vi "DetectorTest_MainV1.vi"() -> ()   [LabVIEW 2012]
uses:
  <vilib>/Analysis/NI_AALBase.lvlib
panel:
  in  "Move to 0 0":bool
  in  "Wafer Info Flash 2":T1={"Cell Name"="5500_130_05", "Package"="", "Coating"="", "LRC?"=enum."J2", "Comment"=""}
  in  "Parameters Flash 2":T2 {"Voc" format="%#_4g"; "Isc" format="%#_4g"; "FF" format="%#_4g"; "Imax" format="%#_4g"; "Vmax" format="%#_4g"; "Pmax" format="%#_4g"; "Itest" format="%#_4g"}
  in  "Wafer Info Flash":T1={"Cell Name"="5500_130_05", "Package"="", "Coating"="", "LRC?"=enum."J2", "Comment"=""}
  in  "Parameters Flash":T2 {"Voc" format="%#_4g"; "Isc" format="%#_4g"; "FF" format="%#_4g"; "Imax" format="%#_4g"; "Vmax" format="%#_4g"; "Pmax" format="%#_4g"; "Itest" format="%#_4g"}
  out "RawData file":path
  out "Fine Cell Clusters":T3(array[cluster])
  out "Selected Data":cluster{dbl[], dbl[]}
  in  "Test Results 2":T4
  in  "Session Info 2":T5={"V set"=-1.0, "I compliance"=0.001, "J set"=0.01, "I set"=0.0, "V compliance"=1.0, "Laser Power (mW)"=0.0, "TestID"=0, "Session Time"=timestamp(0 s since 1904-01-01), "Operator"="Radek"} {"V compliance" format="%#_6f"; "I compliance" format="%#_6e"}
  in  "Die Info 2":T6={"Device Name"="", "ActiveArea_um2"=3848.451, "MesaArea_um2"=3848.451, "x"=0.0, "y"=0.0}
  in  "Wafer Info 2":T7
  in  "Test Results":T4
  in  "Session Info":T5={"V set"=-1.0, "I compliance"=0.001, "J set"=0.01, "I set"=0.0, "V compliance"=1.0, "Laser Power (mW)"=0.0, "TestID"=0, "Session Time"=timestamp(0 s since 1904-01-01), "Operator"="Radek"} {"V compliance" format="%#_6f"; "I compliance" format="%#_6e"}
  in  "Die Info":T6={"Device Name"="", "ActiveArea_um2"=3848.451, "MesaArea_um2"=3848.451, "x"=0.0, "y"=0.0}
  in  "Wafer Info":T7
  in  "Name Array":string[](array[string])=["Wafer name", "Scribe", "Mask", "Lot", "Device name", "Active Area", "Mesa Area", "x", "y", "Imeas", "Vmeas", "Time", "Vset", "Icomp", "Jset", "Iset", "Vcomp", "Laser Power", "TestID", "SessionTime", "Operator", "Selected"]
  in  "TestID file":path=path "C:/Users/Flash/Desktop/LabVIEW/Detector IV/rawtest_log.csv"
  in  "update wafer":bool
  in  "Lot":string
  in  "Laser Power (mW)":dbl
  in  "Device Name":string
  in  "Scribe":string
  in  "MesaArea_um2":dbl=3848.451
  out "Status":string
  out "error out":errorcluster
  in  "error in (no error)":errorcluster
  out "Manaul Plot 1":cluster{"V manual":dbl[], dbl[]}[](array[cluster])
  out "Manual Plot 0":cluster{"V manual":dbl[], "I manual":dbl[]}[](array[cluster])
  in  "Reset 1st die":bool
  in  "Sweep Settings":T8={"Channel"=enum."Channel A", "Vstart"=-2.0, "Vend"=0.5, "# of points"=30, "NPLC"=1.0, "I compliance"=0.001, "Delay ms"=500.0}
  in  "Reset xy":bool
  out "current y":i32
  out "current x":i32
  in  "sweep delay ms":dbl=500.0
  in  "I compliance":dbl=0.001
  in  "points":u16=40
  in  "V end":dbl=0.4
  in  "V start":dbl=-1.5
  in  "Repeat Vf":u32=1
  out "I set":dbl
  in  "V compliance":dbl=1.0 format="%#_6f"
  in  "Vf delay ms":dbl=100.0
  in  "J set A/cm2":dbl=0.01
  in  "Repeat Id":u32=5
  in  "I compliance":dbl=0.001 format="%#_6e"
  in  "Id delay ms":dbl=500.0
  in  "V set":dbl=-1.0
  out "Vmeas Settings":T9={"Channel"=enum."Channel A", "Iset"=-1.0, "NPLC"=1.0, "V compliance"=0.001, "Repeat time"=3, "Delay ms"=500.0}
  out "Imeas Settings":T10={"Channel"=enum."Channel A", "Vset"=-1.0, "NPLC"=1.0, "I compliance"=0.001, "Repeat time"=3, "Delay ms"=500.0}
  out "Array of Cell Data Clusters":T11(array[cluster])=[{"Cell Name"="10000_590_4P5", "X-coord"=0.0, "Y-coord"=0.0, "Area"=110000000.0, "Grid Shadowing"=0.0081, "Ydim"=10000.0, "Xdim"=11000.0, "Meas Area"=0.0}, {"Cell Name"="10000_590_4P5", "X-coord"=10115.0, "Y-coord"=0.0, "Area"=110000000.0, "Grid Shadowing"=0.0081, "Ydim"=10000.0, "Xdim"=11000.0, "Meas Area"=0.0}, {"Cell Name"="10000_590_4P5", "X-coord"=20230.0, "Y-coord"=0.0, "Area"=110000000.0, "Grid Shadowing"=0.0081, "Ydim"=10000.0, "Xdim"=11000.0, "Meas Area"=0.0}, {"Cell Name"="10000_590_4P5", "X-coord"=30345.0, "Y-coord"=0.0, "Area"=110000000.0, "Grid Shadowing"=0.0081, "Ydim"=10000.0, "Xdim"=11000.0, "Meas Area"=0.0}, {"Cell Name"="10000_590_4P5", "X-coord"=-10115.0, "Y-coord"=11515.0, "Area"=110000000.0, "Grid Shadowing"=0.0081, "Ydim"=10000.0, "Xdim"=11000.0, "Meas Area"=0.0}, {"Cell Name"="10000_590_4P5", "X-coord"=0.0, "Y-coord"=11515.0, "Area"=110000000.0, "Grid Shadowing"=0.0081, "Ydim"=10000.0, "Xdim"=11000.0, "Meas Area"=0.0}, {"Cell Name"="10000_590_4P5", "X-coord"=10115.0, "Y-coord"=11515.0, "Area"=110000000.0, "Grid Shadowing"=0.0081, "Ydim"=10000.0, "Xdim"=11000.0, "Meas Area"=0.0}, {"Cell Name"="10000_590_4P5", "X-coord"=20230.0, "Y-coord"=11515.0, "Area"=110000000.0, "Grid Shadowing"=0.0081, "Ydim"=10000.0, "Xdim"=11000.0, "Meas Area"=0.0}, {"Cell Name"="10000_590_4P5", "X-coord"=30345.0, "Y-coord"=11515.0, "Area"=110000000.0, "Grid Shadowing"=0.0081, "Ydim"=10000.0, "Xdim"=11000.0, "Meas Area"=0.0}, {"Cell Name"="10000_590_4P5", "X-coord"=40460.0, "Y-coord"=11515.0, "Area"=110000000.0, "Grid Shadowing"=0.0081, "Ydim"=10000.0, "Xdim"=11000.0, "Meas Area"=0.0}, {"Cell Name"="10000_590_4P5", "X-coord"=-20230.0, "Y-coord"=23030.0, "Area"=110000000.0, "Grid Shadowing"=0.0081, "Ydim"=10000.0, "Xdim"=11000.0, "Meas Area"=0.0}, {"Cell Name"="10000_590_4P5", "X-coord"=-10115.0, "Y-coord"=23030.0, "Area"=110000000.0, "Grid Shadowing"=0.0081, "Ydim"=10000.0, "Xdim"=11000.0, "Meas Area"=0.0}, {"Cell Name"="10000_590_4P5", "X-coord"=0.0, "Y-coord"=23030.0, "Area"=110000000.0, "Grid Shadowing"=0.0081, "Ydim"=10000.0, "Xdim"=11000.0, "Meas Area"=0.0}, {"Cell Name"="10000_590_4P5", "X-coord"=10115.0, "Y-coord"=23030.0, "Area"=110000000.0, "Grid Shadowing"=0.0081, "Ydim"=10000.0, "Xdim"=11000.0, "Meas Area"=0.0}, {"Cell Name"="10000_590_4P5", "X-coord"=20230.0, "Y-coord"=23030.0, "Area"=110000000.0, "Grid Shadowing"=0.0081, "Ydim"=10000.0, "Xdim"=11000.0, "Meas Area"=0.0}, {"Cell Name"="10000_590_4P5", "X-coord"=30345.0, "Y-coord"=23030.0, "Area"=110000000.0, "Grid Shadowing"=0.0081, "Ydim"=10000.0, "Xdim"=11000.0, "Meas Area"=0.0}, {"Cell Name"="10000_590_4P5", "X-coord"=40460.0, "Y-coord"=23030.0, "Area"=110000000.0, "Grid Shadowing"=0.0081, "Ydim"=10000.0, "Xdim"=11000.0, "Meas Area"=0.0}, {"Cell Name"="10000_590_4P5", "X-coord"=50575.0, "Y-coord"=23030.0, "Area"=110000000.0, "Grid Shadowing"=0.0081, "Ydim"=10000.0, "Xdim"=11000.0, "Meas Area"=0.0}, {"Cell Name"="10000_590_4P5", "X-coord"=-20230.0, "Y-coord"=34545.0, "Area"=110000000.0, "Grid Shadowing"=0.0081, "Ydim"=10000.0, "Xdim"=11000.0, "Meas Area"=0.0}, {"Cell Name"="10000_590_4P5", "X-coord"=-10115.0, "Y-coord"=34545.0, "Area"=110000000.0, "Grid Shadowing"=0.0081, "Ydim"=10000.0, "Xdim"=11000.0, "Meas Area"=0.0}, {"Cell Name"="10000_590_4P5", "X-coord"=0.0, "Y-coord"=34545.0, "Area"=110000000.0, "Grid Shadowing"=0.0081, "Ydim"=10000.0, "Xdim"=11000.0, "Meas Area"=0.0}, {"Cell Name"="10000_590_4P5", "X-coord"=10115.0, "Y-coord"=34545.0, "Area"=110000000.0, "Grid Shadowing"=0.0081, "Ydim"=10000.0, "Xdim"=11000.0, "Meas Area"=0.0}, {"Cell Name"="10000_590_4P5", "X-coord"=20230.0, "Y-coord"=34545.0, "Area"=110000000.0, "Grid Shadowing"=0.0081, "Ydim"=10000.0, "Xdim"=11000.0, "Meas Area"=0.0}, {"Cell Name"="10000_590_4P5", "X-coord"=30345.0, "Y-coord"=34545.0, "Area"=110000000.0, "Grid Shadowing"=0.0081, "Ydim"=10000.0, "Xdim"=11000.0, "Meas Area"=0.0}, {"Cell Name"="10000_590_4P5", "X-coord"=40460.0, "Y-coord"=34545.0, "Area"=110000000.0, "Grid Shadowing"=0.0081, "Ydim"=10000.0, "Xdim"=11000.0, "Meas Area"=0.0}, {"Cell Name"="10000_590_4P5", "X-coord"=50575.0, "Y-coord"=34545.0, "Area"=110000000.0, "Grid Shadowing"=0.0081, "Ydim"=10000.0, "Xdim"=11000.0, "Meas Area"=0.0}, {"Cell Name"="10000_590_4P5", "X-coord"=-20230.0, "Y-coord"=46060.0, "Area"=110000000.0, "Grid Shadowing"=0.0081, "Ydim"=10000.0, "Xdim"=11000.0, "Meas Area"=0.0}, {"Cell Name"="10000_590_4P5", "X-coord"=-10115.0, "Y-coord"=46060.0, "Area"=110000000.0, "Grid Shadowing"=0.0081, "Ydim"=10000.0, "Xdim"=11000.0, "Meas Area"=0.0}, {"Cell Name"="10000_590_4P5", "X-coord"=0.0, "Y-coord"=46060.0, "Area"=110000000.0, "Grid Shadowing"=0.0081, "Ydim"=10000.0, "Xdim"=11000.0, "Meas Area"=0.0}, {"Cell Name"="10000_590_4P5", "X-coord"=10115.0, "Y-coord"=46060.0, "Area"=110000000.0, "Grid Shadowing"=0.0081, "Ydim"=10000.0, "Xdim"=11000.0, "Meas Area"=0.0}, {"Cell Name"="10000_590_4P5", "X-coord"=20230.0, "Y-coord"=46060.0, "Area"=110000000.0, "Grid Shadowing"=0.0081, "Ydim"=10000.0, "Xdim"=11000.0, "Meas Area"=0.0}, {"Cell Name"="10000_590_4P5", "X-coord"=30345.0, "Y-coord"=46060.0, "Area"=110000000.0, "Grid Shadowing"=0.0081, "Ydim"=10000.0, "Xdim"=11000.0, "Meas Area"=0.0}, {"Cell Name"="10000_590_4P5", "X-coord"=40460.0, "Y-coord"=46060.0, "Area"=110000000.0, "Grid Shadowing"=0.0081, "Ydim"=10000.0, "Xdim"=11000.0, "Meas Area"=0.0}, {"Cell Name"="10000_590_4P5", "X-coord"=50575.0, "Y-coord"=46060.0, "Area"=110000000.0, "Grid Shadowing"=0.0081, "Ydim"=10000.0, "Xdim"=11000.0, "Meas Area"=0.0}, {"Cell Name"="10000_590_4P5", "X-coord"=-10115.0, "Y-coord"=57575.0, "Area"=110000000.0, "Grid Shadowing"=0.0081, "Ydim"=10000.0, "Xdim"=11000.0, "Meas Area"=0.0}, {"Cell Name"="10000_590_4P5", "X-coord"=0.0, "Y-coord"=57575.0, "Area"=110000000.0, "Grid Shadowing"=0.0081, "Ydim"=10000.0, "Xdim"=11000.0, "Meas Area"=0.0}, {"Cell Name"="10000_590_4P5", "X-coord"=10115.0, "Y-coord"=57575.0, "Area"=110000000.0, "Grid Shadowing"=0.0081, "Ydim"=10000.0, "Xdim"=11000.0, "Meas Area"=0.0}, {"Cell Name"="10000_590_4P5", "X-coord"=20230.0, "Y-coord"=57575.0, "Area"=110000000.0, "Grid Shadowing"=0.0081, "Ydim"=10000.0, "Xdim"=11000.0, "Meas Area"=0.0}, {"Cell Name"="10000_590_4P5", "X-coord"=30345.0, "Y-coord"=57575.0, "Area"=110000000.0, "Grid Shadowing"=0.0081, "Ydim"=10000.0, "Xdim"=11000.0, "Meas Area"=0.0}, {"Cell Name"="10000_590_4P5", "X-coord"=40460.0, "Y-coord"=57575.0, "Area"=110000000.0, "Grid Shadowing"=0.0081, "Ydim"=10000.0, "Xdim"=11000.0, "Meas Area"=0.0}, {"Cell Name"="10000_590_4P5", "X-coord"=0.0, "Y-coord"=69090.0, "Area"=110000000.0, "Grid Shadowing"=0.0081, "Ydim"=10000.0, "Xdim"=11000.0, "Meas Area"=0.0}, {"Cell Name"="10000_590_4P5", "X-coord"=10115.0, "Y-coord"=69090.0, "Area"=110000000.0, "Grid Shadowing"=0.0081, "Ydim"=10000.0, "Xdim"=11000.0, "Meas Area"=0.0}, {"Cell Name"="10000_590_4P5", "X-coord"=20230.0, "Y-coord"=69090.0, "Area"=110000000.0, "Grid Shadowing"=0.0081, "Ydim"=10000.0, "Xdim"=11000.0, "Meas Area"=0.0}, {"Cell Name"="10000_590_4P5", "X-coord"=30345.0, "Y-coord"=69090.0, "Area"=110000000.0, "Grid Shadowing"=0.0081, "Ydim"=10000.0, "Xdim"=11000.0, "Meas Area"=0.0}]
  in  "stop":bool
  in  "ActiveArea_um2":dbl=3848.451
  in  "NPLC":dbl=1.0
  in  "Operator":string(combo)="Radek"
  in  "Mask":string
  in  "Wafer Name":string
  in  "Tab Control":T12(tab)
  in  "Manual_Test":bool
  in  "Manual IV settting":enum32{"Linear plot", "Log plot"}(radio)
  out "Vmeas manual":dbl
  out "Imeas manual":dbl
  out "Iarray manual":dbl[](array[numeric])
  out "Varray manual":dbl[](array[numeric])
  out "y target":i32
  out "x target":i32
  in  "Die Number":u16(ring) items=["0", "1", "2", "3", "4", "5", "6", "7", "8", "9"]
  in  "load file":bool
  in  "Move to":bool
  in  "Mask File Manual":path=path "C:/Users/Flash/Desktop/Mask Files/SL066 Detector/SL066_D5_20_align on D3000.csv"
  out "Manual IV":cluster{"V manual":dbl[], "I manual":dbl[]}[](graph)
  in  "Load raw":bool
  in  "Select":bool
  in  "Number Select":u16=10
  in  "Vmax":dbl=0.95
  in  "Vmin":dbl
  out "Test FileName":string
  out "RawTest ID":u32
  out "Progress":u8(slide) scale=0.0..100.0
  out "Current Device":u32
  out "Total Device":u32
  out "V meas":dbl[](array[numeric])
  out "I meas":dbl[](array[numeric])
  in  "RawData Save Path":path=path "C:/Users/Flash/Desktop/Data/Detector test data"
  in  "StartRaw":bool
  out "Vforward hist":T13(graph)
  out "Idark hist":T13(graph)
  in  "Mask File Raw":path=path "C:/Users/Flash/Desktop/Mask Files/SL066 Detector/SL066_D5_20_align on D3000.csv"
  out "Spec Plot":cluster{"V meas":dbl[], "I meas":dbl[]}[](graph)
  in  "Auto Select and Fine Test?":bool
  in  "FineTest save path":path=path "C:/Users/Flash/Desktop/Data/Detector test data/IV"
  out "I fine":dbl[](array[numeric])
  out "V fine":dbl[](array[numeric])
  out "Current Device":u32
  out "Total Device":u32
  out "IV fine log":cluster{dbl[], dbl[]}[](graph)
  out "Progress 2":u8(slide) scale=0.0..100.0
  in  "StartFine":bool
  out "IV fine linear":cluster{dbl[], dbl[]}[](graph)
  in  "Mask File Fine":path=path "C:/Users/Flash/Desktop/Mask Files/SL066 Detector/SL066_D5_20_align on D3000.csv"
  in  "Prober GPIB":string="0:1"
  in  "SMU":refnum<visa-resource-name>="GPIB0::26::INSTR"
  in  "Channel":enum32{"Channel A", "Channel B"}(ring)
  # "0 is for dark IV!"
  # "Sweep Settings"
  # "Forward Voltage"
  # "Dark/Light Current"
  # "Make sure current x and y are same as prober before click Start!"
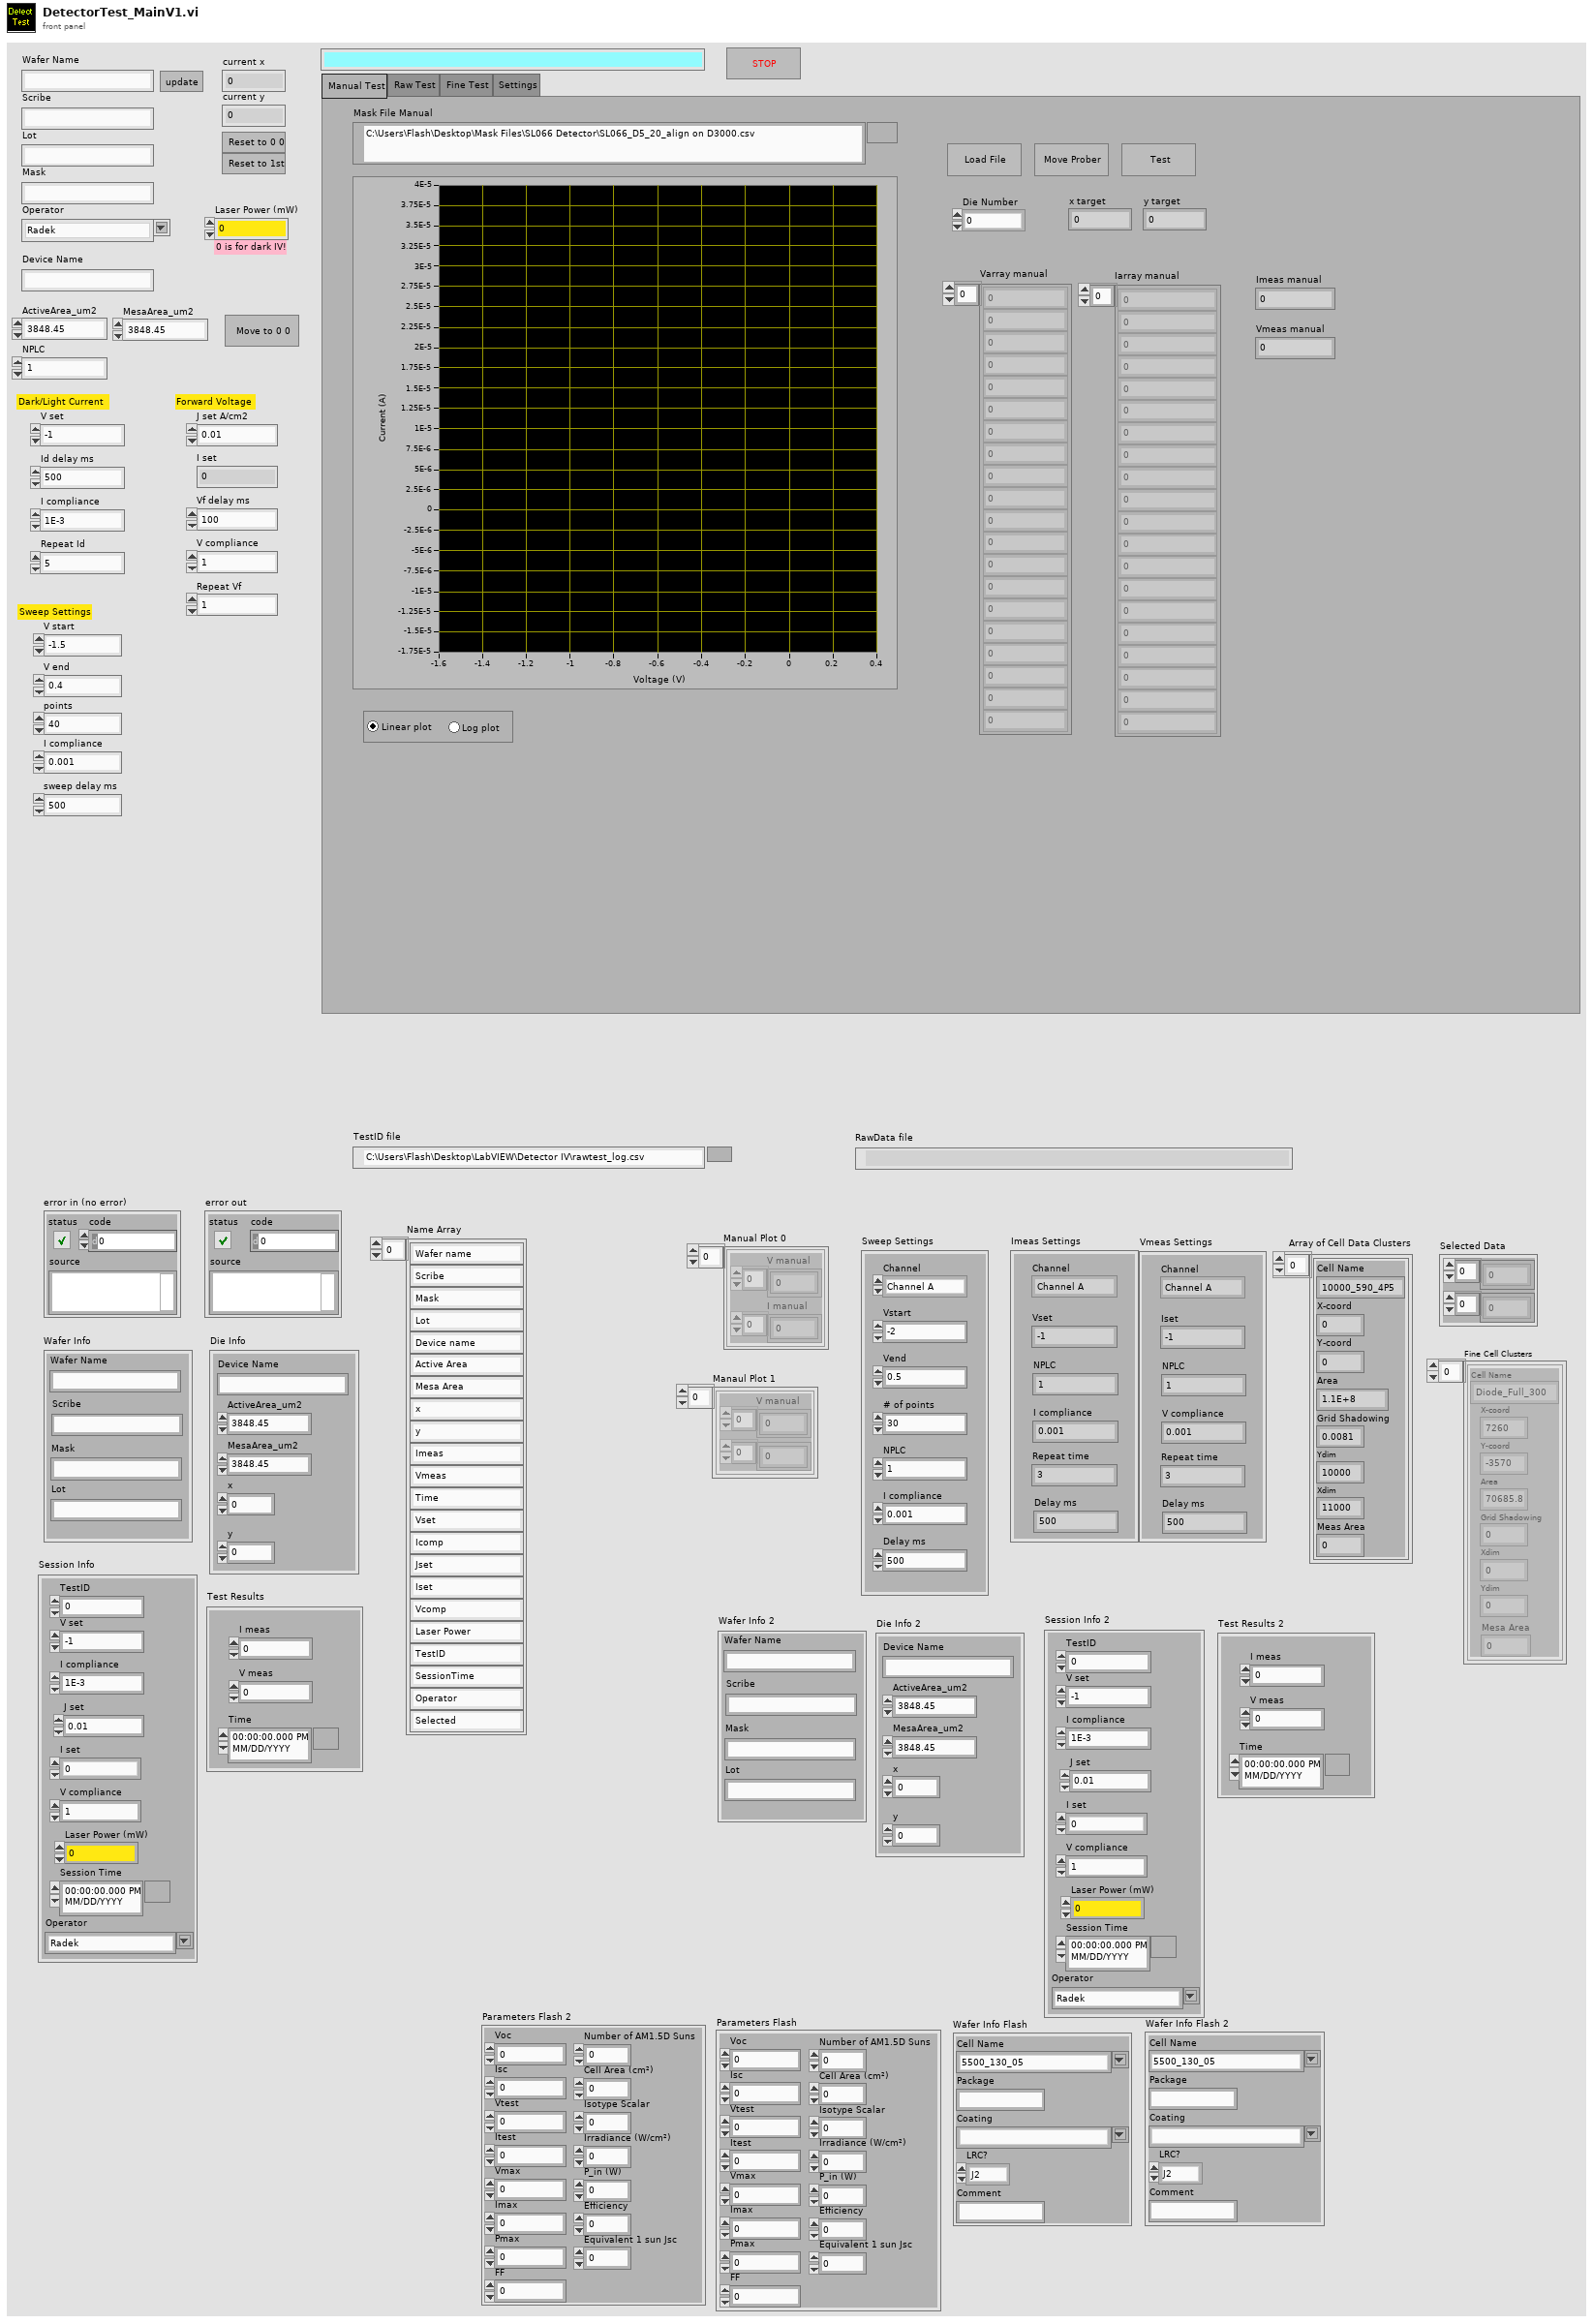
[diagram p1: front panel]
types:
  T1 = cluster{"Cell Name":string, "Package":string, "Coating":string, "LRC?":enum16{"J1", "J2", "LRC"}, "Comment":string}
  T2 = cluster{"Voc":dbl, "Isc":dbl, "FF":dbl, "Vtest":dbl, "Imax":dbl, "Vmax":dbl, "Pmax":dbl, "Itest":dbl, "Efficiency":dbl, "P_in (W)":dbl, "Irradiance (W/cm²)":dbl, "Cell Area (cm²)":dbl, "Number of AM1.5D Suns":dbl, "Isotype Scalar":dbl, "Equivalent 1 sun Jsc":dbl}
  T3 = cluster{"Cell Name":string, "X-coord":dbl, "Y-coord":dbl, "Area":dbl, "Grid Shadowing":dbl, "Xdim":dbl, "Ydim":dbl, "Mesa Area":dbl}[]
  T4 = cluster{"I meas":dbl, "V meas":dbl, "Time":timestamp}
  T5 = cluster{"V set":dbl, "I compliance":dbl, "J set":dbl, "I set":dbl, "V compliance":dbl, "Laser Power (mW)":dbl, "TestID":u32, "Session Time":timestamp, "Operator":string}
  T6 = cluster{"Device Name":string, "ActiveArea_um2":dbl, "MesaArea_um2":dbl, "x":dbl, "y":dbl}
  T7 = cluster{"Wafer Name":string, "Scribe":string, "Mask":string, "Lot":string}
  T8 = cluster{"Channel":enum32{"Channel A", "Channel B"}, "Vstart":dbl, "Vend":dbl, "# of points":u16, "NPLC":dbl, "I compliance":dbl, "Delay ms":dbl}
  T9 = cluster{"Channel":enum32{"Channel A", "Channel B"}, "Iset":dbl, "NPLC":dbl, "V compliance":dbl, "Repeat time":u16, "Delay ms":dbl}
  T10 = cluster{"Channel":enum32{"Channel A", "Channel B"}, "Vset":dbl, "NPLC":dbl, "I compliance":dbl, "Repeat time":u16, "Delay ms":dbl}
  T11 = cluster{"Cell Name":string, "X-coord":dbl, "Y-coord":dbl, "Area":dbl, "Grid Shadowing":dbl, "Ydim":dbl, "Xdim":dbl, "Meas Area":dbl}[]
  T12 = enum32{"Manual Test", "Raw Test", "Fine Test", "Settings"}
  T13 = cluster{"X Values":dbl[], "Histogram: h(x)":i32[]}
  T14 = cluster{"Cell Name":string, "X-coord":dbl, "Y-coord":dbl, "Area":dbl, "Grid Shadowing":dbl, "Ydim":dbl, "Xdim":dbl, "Meas Area":dbl}
  T15 = cluster{"Varray manual":dbl[], "Iarray manual":dbl[]}[]
  T16 = cluster{"WaferName":string, "Scribe":string, "Structure":string, "Lot":string, "Mask":string}
  T17 = cluster{"V set":dbl, "I compliance":dbl, "J set":dbl, "I set":dbl, "V compliance":dbl, "Laser Power (mW)":dbl, "TestID":u32, "Operator":string}
  T18 = cluster{"Device Name":string, "ActiveArea_um2":dbl, "MesaArea_um2":dbl}
  T19 = cluster{"Cell Name":string, "X-coord":dbl, "Y-coord":dbl, "Area":dbl, "Grid Shadowing":dbl, "Xdim":dbl, "Ydim":dbl, "Mesa Area":dbl}
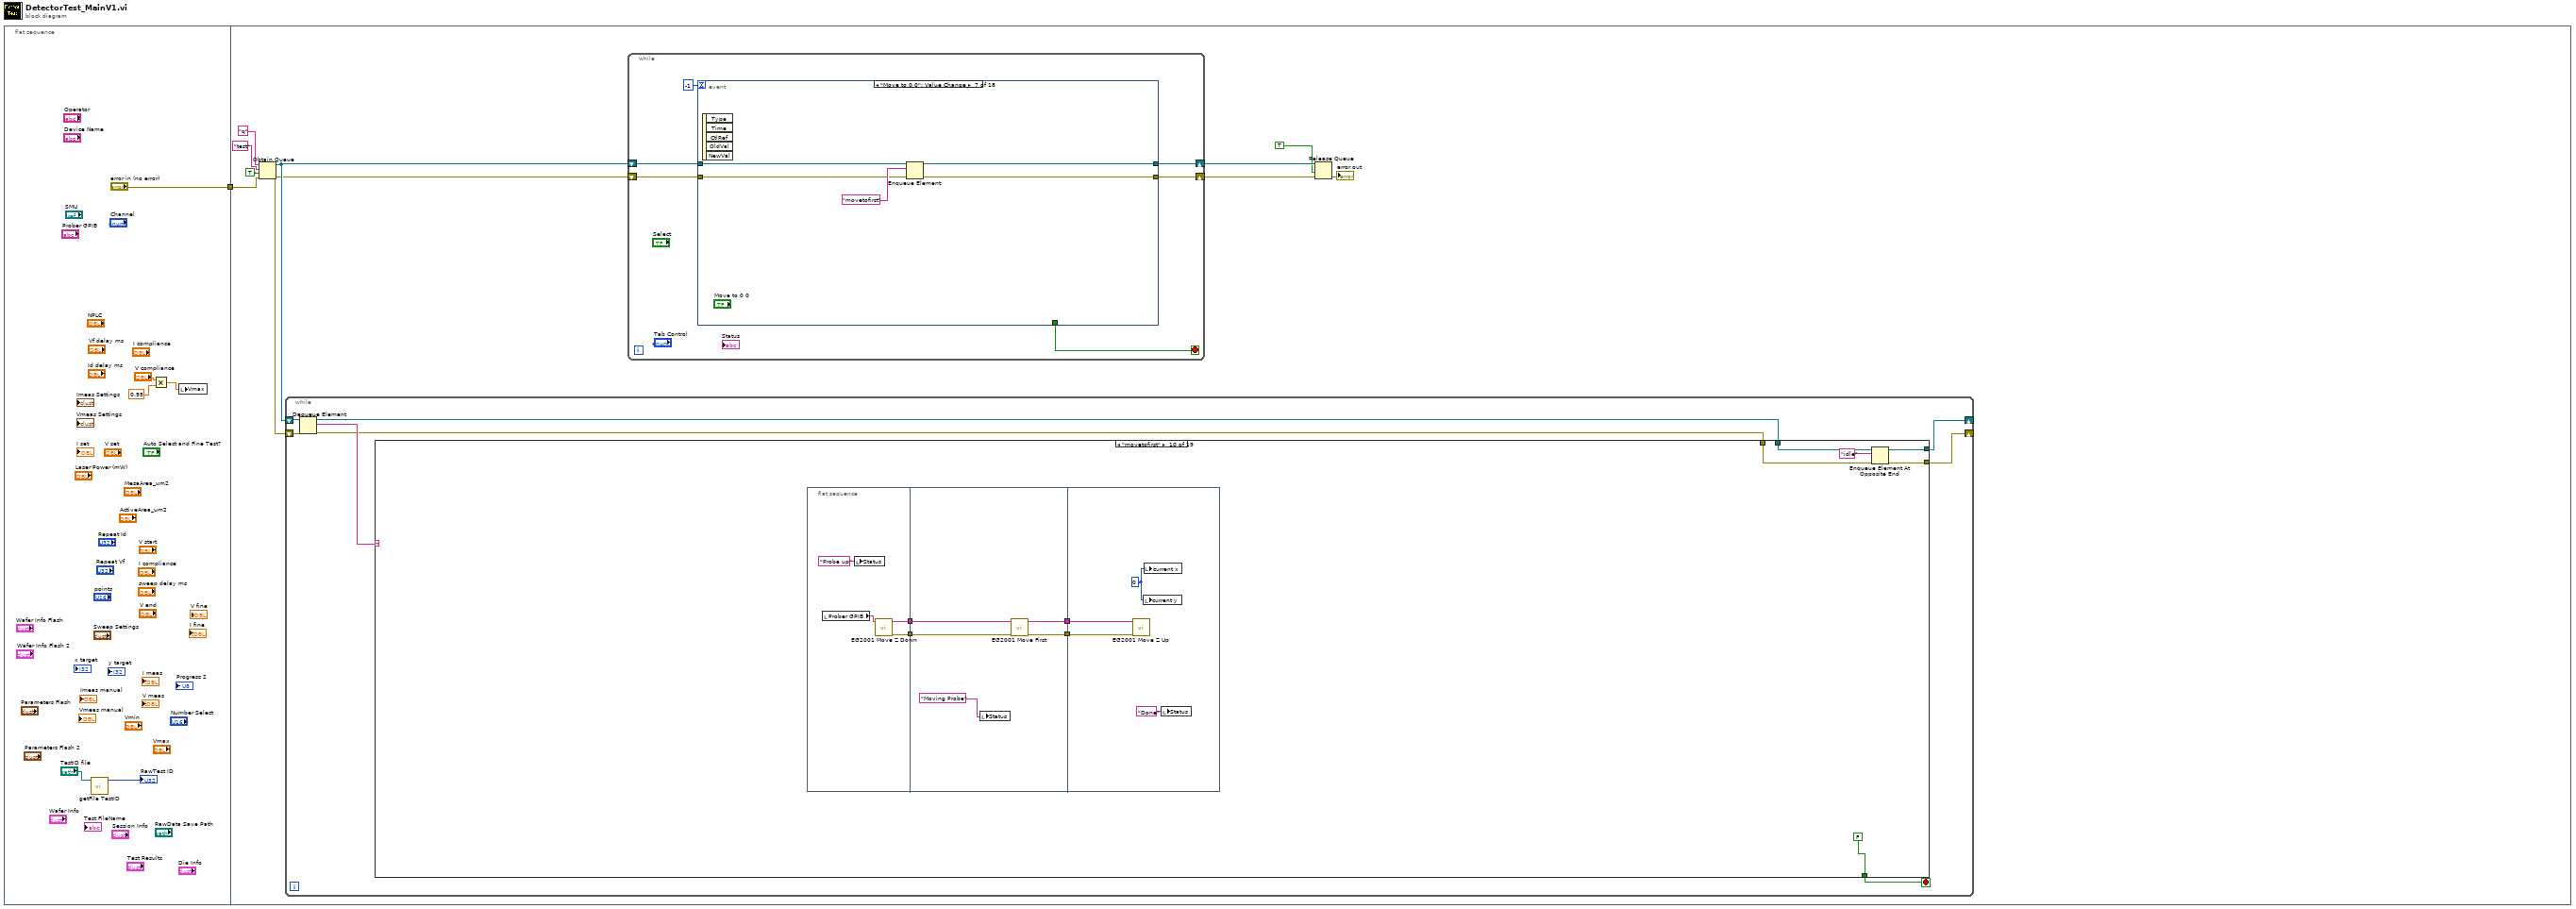
[diagram p0: block diagram]
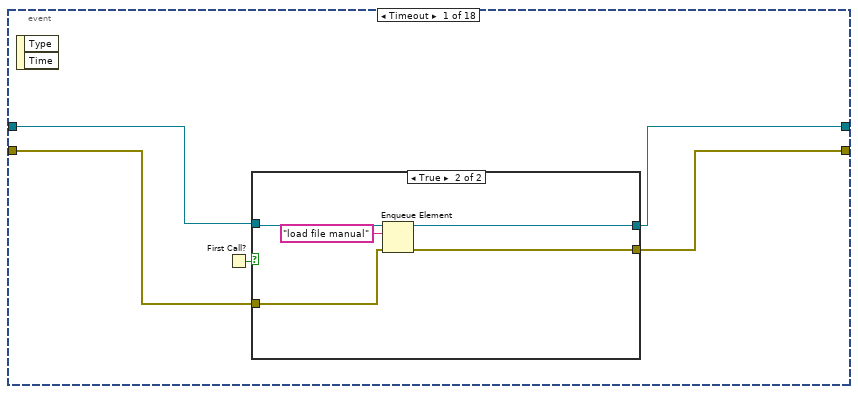
[diagram p2: hidden frame]
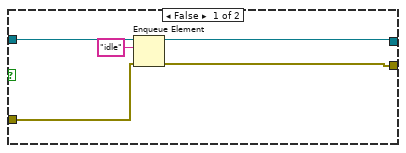
[diagram p3: hidden frame]
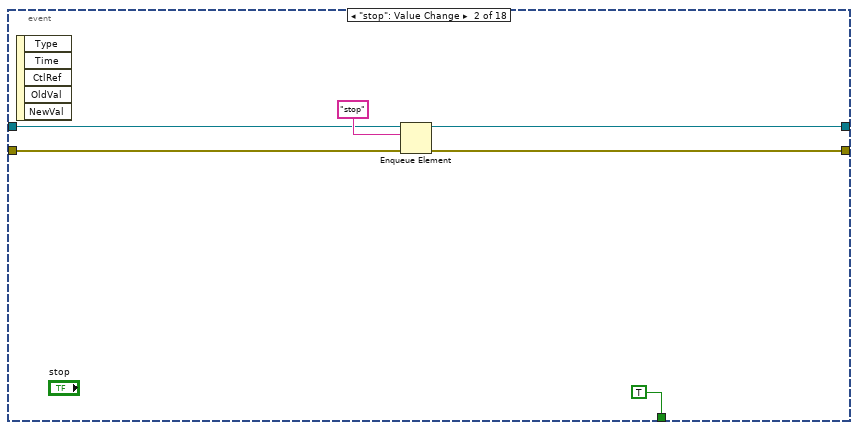
[diagram p4: hidden frame]
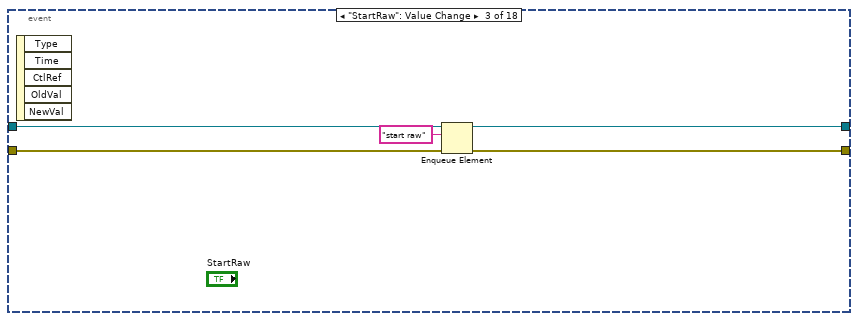
[diagram p5: hidden frame]
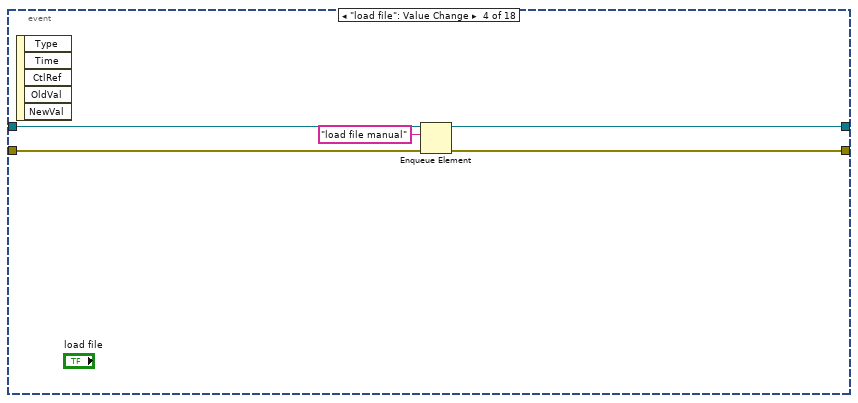
[diagram p6: hidden frame]
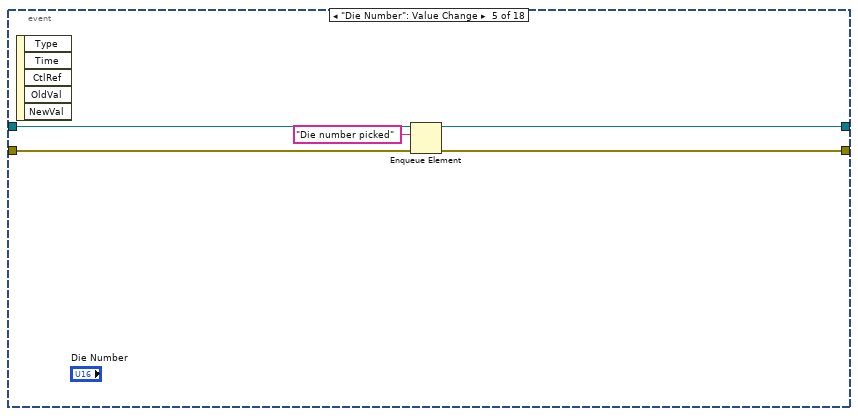
[diagram p7: hidden frame]
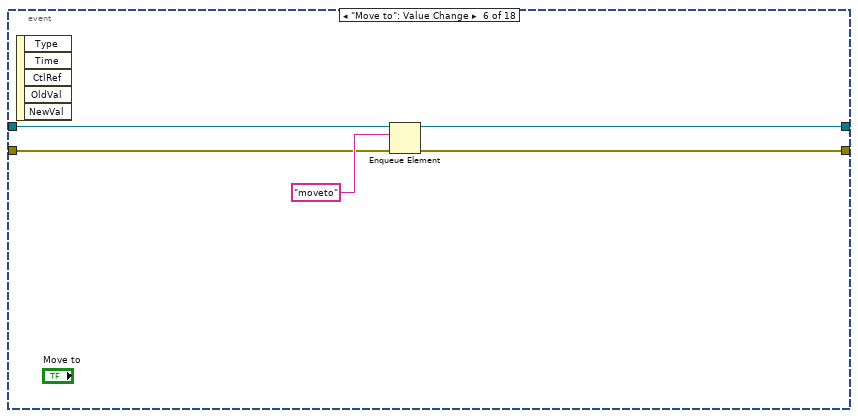
[diagram p8: hidden frame]
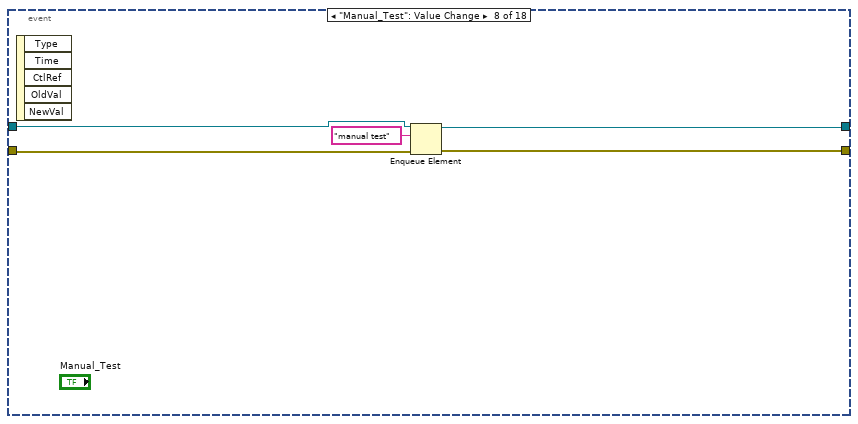
[diagram p9: hidden frame]
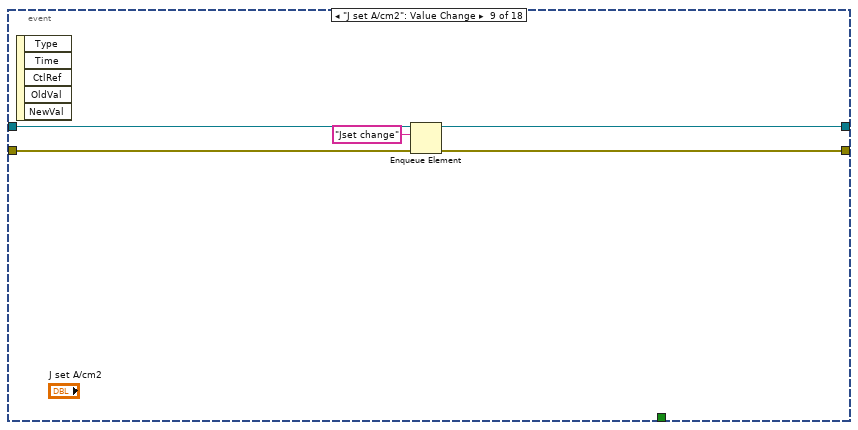
[diagram p10: hidden frame]
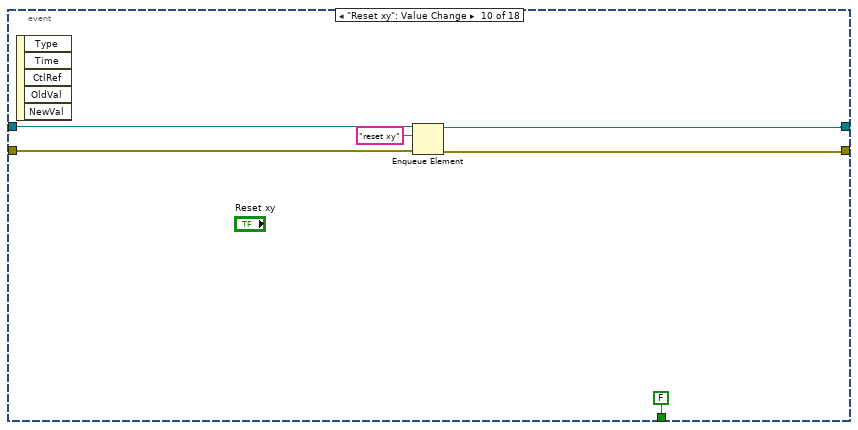
[diagram p11: hidden frame]
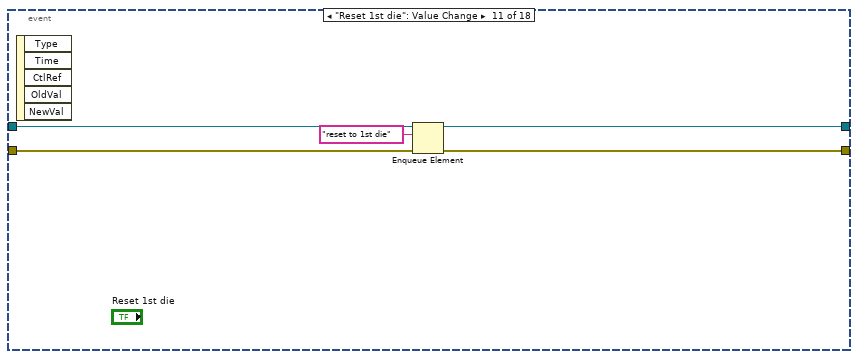
[diagram p12: hidden frame]
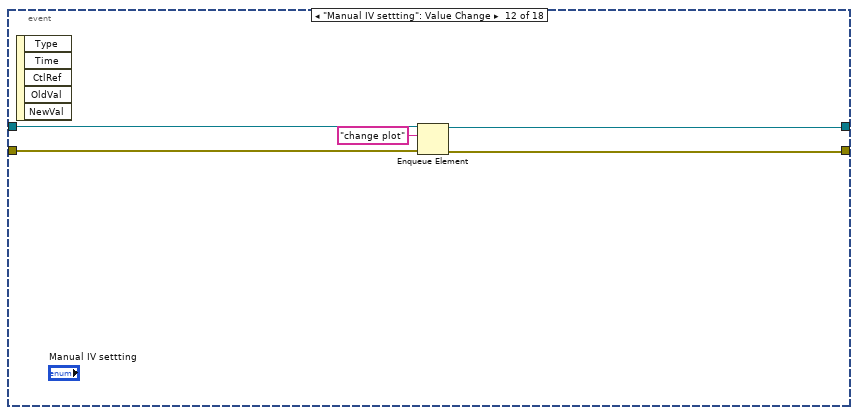
[diagram p13: hidden frame]
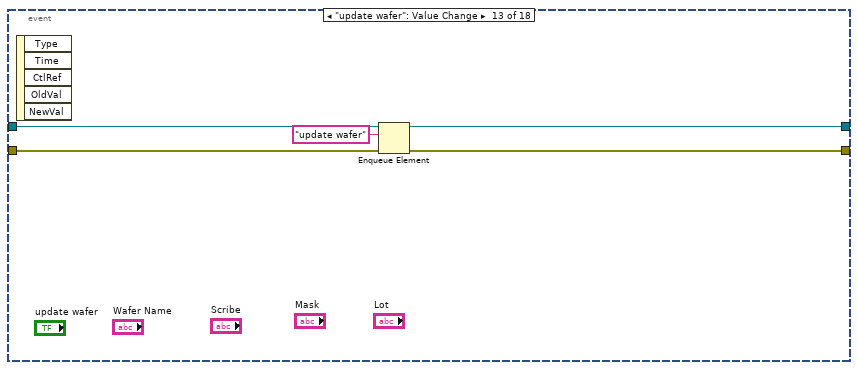
[diagram p14: hidden frame]
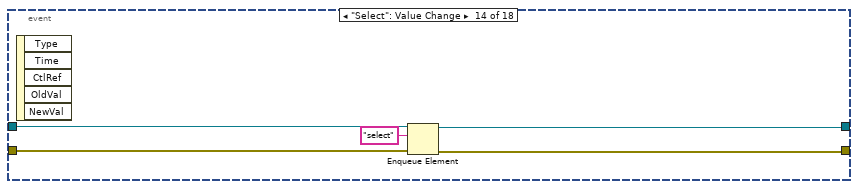
[diagram p15: hidden frame]
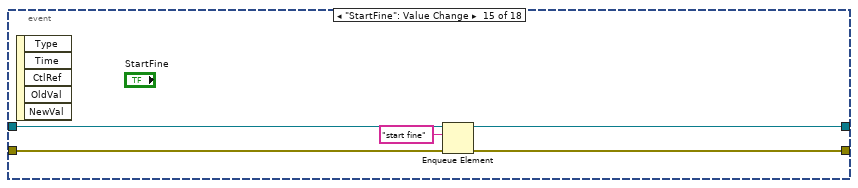
[diagram p16: hidden frame]
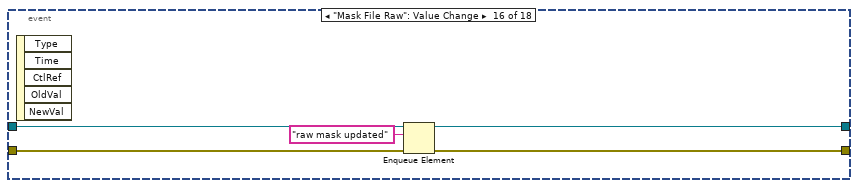
[diagram p17: hidden frame]
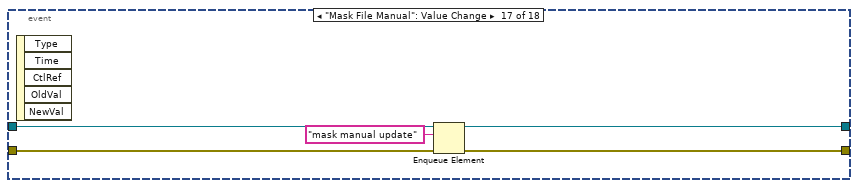
[diagram p18: hidden frame]
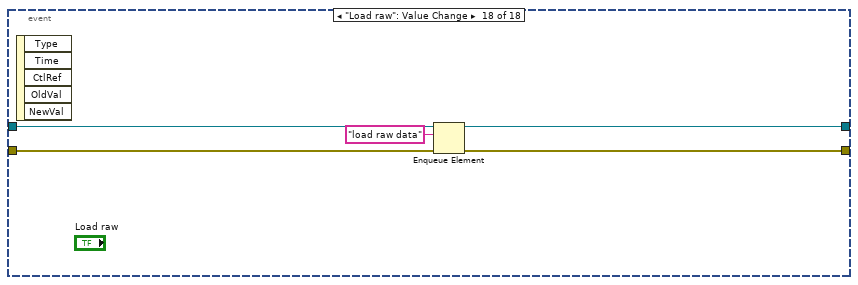
[diagram p19: hidden frame]
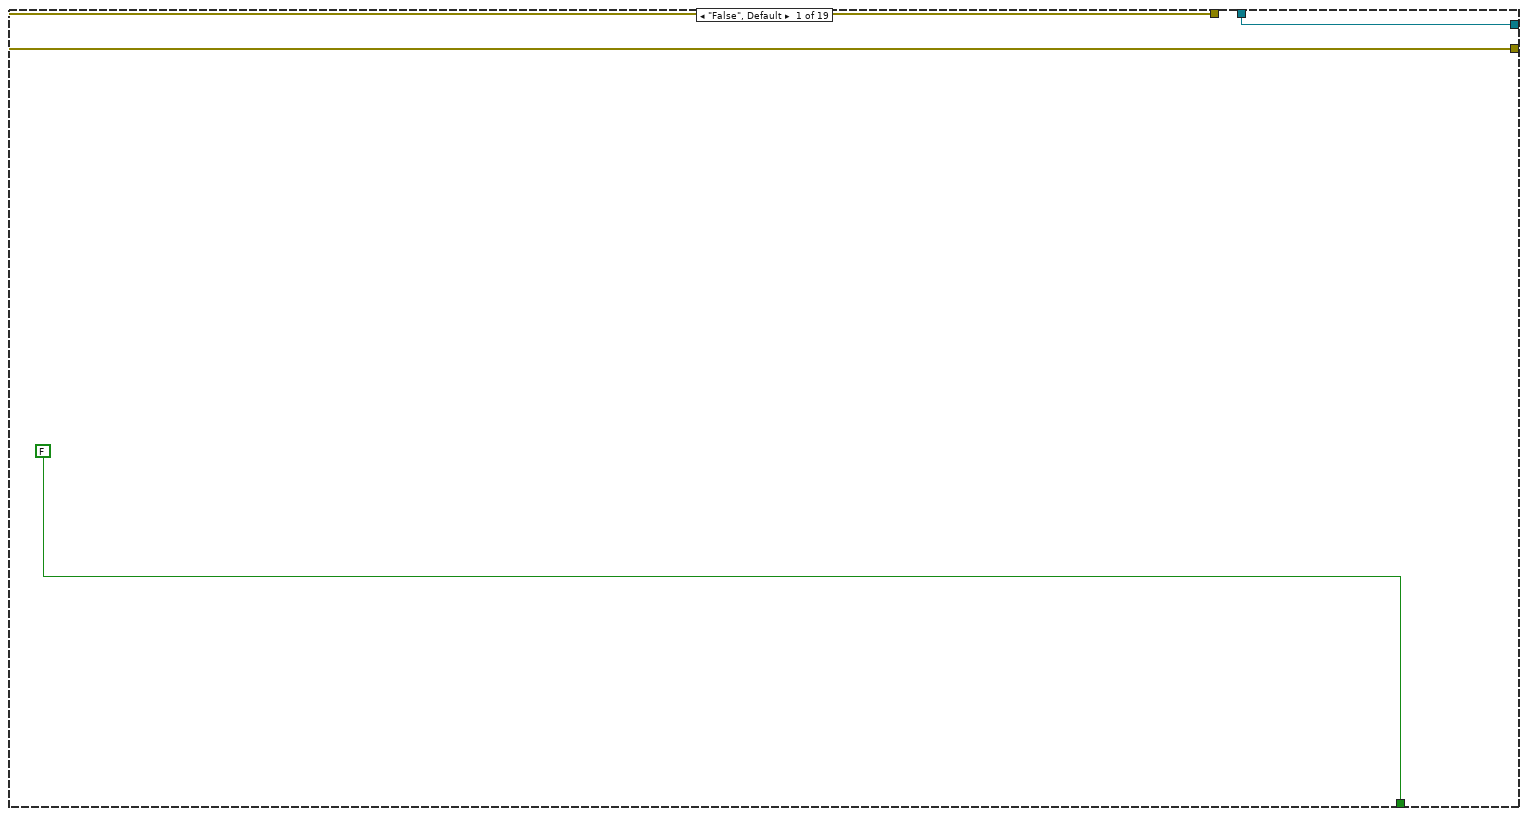
[diagram p20: hidden frame]
diagram:
  n1 = flat-sequence {
    tunnel: ["error in (no error)"] -> w1
    tunnel: w1 -> [w14]
    frame #0 {
      n2 = call "getFile TestID.vi"("Path"="TestID file") -> ("TestID"=→"RawTest ID":u32)  [unwired: 9 in, 1 out]
      n3 = Multiply(x="V compliance", y=0.95) -> (x*y=w2:dbl)
      n4 = local write "Vmax"(w2) -> ()
    }
    frame #1 {
      n5 = Obtain Queue(name (unnamed)="q", element data type="test" ("name (unnamed)"), create if not found? (T)=TRUE, error in (no error)=w14) -> (queue out=w16:refnum<queue>, error out=w15:errorcluster)  [unwired: 1 in, 1 out]
      n6 = while {
        shift-right: [w131] -> _
        shift-left: w16 -> [w128]
        shift-right: [w130] -> _
        shift-left: w15 -> [w127]
        stop <- w133 stop-if-true
        n7 = Dequeue Element(queue=w128, error in (no error)=w127) -> (queue out=w126:refnum<queue>, element=w132:string, error out=w129:errorcluster)  [unwired: 1 in, 1 out]
        n8 = case shown="\"movetofirst\"" w132 {
          tunnel: [FALSE TRUE FALSE FALSE FALSE FALSE FALSE FALSE FALSE FALSE FALSE FALSE FALSE FALSE FALSE FALSE FALSE FALSE FALSE] -> w133
          tunnel: w129 -> [w135 w138 w143 w303 w314 w325 w356 w380 w393 w425 w450 w530 w540 w547 w562 w597 w634 w775 w786]
          tunnel: [w135 w138 w144 w304 w311 w322 w359 w381 w396 w428 w449 w535 w540 w546 w564 w599 w636 w777 w788] -> w130
          tunnel: w126 -> [w134 w137 w146 w306 w313 w324 w357 w383 w398 w430 w447 w537 w541 w545 w563 w598 w635 w776 w787]
          tunnel: [w134 w137 w145 w305 w312 w323 w358 w382 w397 w429 w448 w536 w541 w544 w565 w600 w637 w778 w789] -> w131
          frame "False", Default {
          }
          frame "stop" {
          }
          frame "start raw" {
            n9 = flat-sequence {
              tunnel: [w157] -> w142
              tunnel: w142 -> [w187]
              tunnel: [w187] -> w141
              tunnel: [w177] -> w140
              tunnel: w141 -> [w189]
              tunnel: w140 -> [w188]
              frame #0 {
                n10 = local read "Wafer Name"() -> (w155:string)
                n11 = local read "RawTest ID"() -> (w160:u32)
                n12 = local read "Scribe"() -> (w154:string)
                n13 = local read "Mask"() -> (w153:string)
                n14 = local read "Lot"() -> (w152:string)
                n15 = call "Device Files v1.vi"("Rows"=1200, "Mask file path"="Mask File Raw") -> ("size(s)"=w157:i32, "Array of Cell Clusters"=→"Array of Cell Data Clusters":T3)  [unwired: 6 in, 2 out]
                "Total Device" <- w157
                n16 = Increment(x=w160) -> (x+1=w159:u32)
                n17 = Bundle By Name(cluster="Wafer Info 2", "Wafer Name"=w155, "Scribe"=w154, "Mask"=w153, "Lot"=w152) -> (w156:T7)
                n18 = local write "Status"("Prepare raw test" ("Status")) -> ()
                n19 = Initialize Array(nan ("element"), w157) -> (w150:dbl[])
                n20 = local write "RawTest ID"(w159) -> ()
                n21 = Bundle(w150, w150) -> (→"Selected Data":cluster{dbl[], dbl[]})  [unwired: 1 in]
                n22 = local write "Wafer Info"(w156) -> ()
                n23 = local write "V meas"(w150) -> ()
                n24 = local write "I meas"(w150) -> ()
                "Progress" <- u8 0 ("Progress")
              }
              frame #1 {
                n25 = local read "Laser Power (mW)"() -> (w168:dbl)
                n26 = local read "V compliance"() -> (w169:dbl)
                n27 = local read "RawData Save Path"() -> (w181:path)
                n28 = local read "I compliance"() -> (w172:dbl)
                n29 = local read "RawTest ID"() -> (w167:u32)
                n30 = local read "Array of Cell Data Clusters"() -> (w186:T11)
                n31 = local read "Operator"() -> (w166:string)
                n32 = local read "J set A/cm2"() -> (w171:dbl)
                n33 = local read "Wafer Name"() -> (w183:string)
                n34 = local read "V set"() -> (w173:dbl)
                n35 = local read "I set"() -> (w170:dbl)
                n36 = Index Array(array=w186, index=0) -> (element=w184:T14)
                n37 = Unbundle By Name(w184) -> ("Cell Name"=w182:string)
                n38 = call "get RawTest filename.vi"("Device Name"=w182, "Wafer Name"=w183) -> ("current time"=w174:timestamp, "FileName"=w180:string)  [unwired: 8 in]
                n39 = Build Path(base path=w181, name or relative path=w180) -> (appended path=w179:path)
                n40 = local write "Test FileName"(w180) -> ()
                n41 = Bundle By Name(cluster="Session Info 2", "V set"=w173, "I compliance"=w172, "J set"=w171, "I set"=w170, "V compliance"=w169, "Laser Power (mW)"=w168, "TestID"=w167, "Session Time"=w174, "Operator"=w166) -> (w175:T5)
                n42 = call "writeFile RawTestHead.vi"("Name Array"="Name Array", "Path"=w179) -> ("Path out"=w177:path)  [unwired: 9 in]
                "RawData file" <- w177
                n43 = local write "Session Info"(w175) -> ()
              }
              frame #2 {
                n44 = for {
                  N: w189 -> [w202]
                  tunnel: w188 -> [w190]
                  i -> [w191]
                  n45 = flat-sequence {
                    tunnel: [w237] -> w212
                    tunnel: [w236] -> w211
                    tunnel: w191 -> [w230]
                    tunnel: [w232] -> w206
                    tunnel: [w231] -> w205
                    tunnel: [w214] -> w204
                    tunnel: [w213] -> w203
                    tunnel: w212 -> [w238]
                    tunnel: w211 -> [w246]
                    tunnel: [w245] -> w210
                    tunnel: [w244] -> w209
                    tunnel: w206 -> [w242]
                    tunnel: w205 -> [w241]
                    tunnel: w204 -> [w240]
                    tunnel: w203 -> [w239]
                    tunnel: w210 -> [w249]
                    tunnel: w209 -> [w248]
                    tunnel: [w259] -> w208
                    tunnel: [w258] -> w207
                    tunnel: w208 -> [w262]
                    tunnel: w207 -> [w270]
                    tunnel: [w262] -> w193
                    tunnel: [w263] -> w192
                    tunnel: w193 -> [w281]
                    tunnel: w192 -> [w280]
                    tunnel: w191 -> [w287]
                    tunnel: w190 -> [w278]
                    frame #0 {
                      n46 = local read "Array of Cell Data Clusters"() -> (w234:T11)
                      n47 = local read "Device Name"() -> (w217:string)
                      n48 = Increment(x=w230) -> (x+1=→"Current Device":i32)
                      n49 = local read "Laser Power (mW)"() -> (w226:dbl)
                      n50 = Index Array(array=w234, index=w230) -> (element=w227:T14)
                      n51 = local read "Prober GPIB"() -> (w228:string)
                      n52 = Unbundle By Name(w227) -> ("X-coord"=w214:dbl, "Y-coord"=w213:dbl, "Area"=w215:dbl, "Meas Area"=w216:dbl, "Cell Name"=w220:string)
                      n53 = Bundle By Name(cluster="Die Info 2", "Device Name"=w217, "ActiveArea_um2"=w215, "MesaArea_um2"=w216, "x"=w214, "y"=w213) -> (w218:T6)
                      n54 = call "get Area.vi"("Laser"=w226, "Cell Data Cluster"=w227) -> ("Area"=w224:dbl)  [unwired: 9 in]
                      n55 = local read "J set A/cm2"() -> (w222:dbl)
                      n56 = local write "ActiveArea_um2"(w215) -> ()
                      n57 = local write "MesaArea_um2"(w216) -> ()
                      n58 = local write "Device Name"(w220) -> ()
                      n59 = Divide(x=w224, y=100000000.0) -> (x/y=w223:dbl)
                      n60 = local read "current y"() -> (w233:i32)
                      n61 = call "EG2001 Move Z Down.vi"("GPIB Address"=w228) -> ("Error Out"=w236:errorcluster, "GPIB Address Out"=w237:string)  [unwired: 9 in]
                      n62 = local read "current x"() -> (w235:i32)
                      n63 = local write "Die Info"(w218) -> ()
                      n64 = Multiply(x=w222, y=w223) -> (x*y=w221:dbl)
                      n65 = local write "I set"(w221) -> ()
                      n66 = Subtract(x=w214, y=w235) -> (x-y=w232:dbl)
                      n67 = Subtract(x=w213, y=w233) -> (x-y=w231:dbl)
                    }
                    frame #1 {
                      n68 = local write "current x"(w240) -> ()
                      n69 = local write "current y"(w239) -> ()
                      n70 = call "EG2001 Move Machine Step X-Y.vi"("Flip X Coordinates?"=FALSE, "Y"=w241, "Steps/Microns"=enum32{"Steps", "Microns"}."Microns", "X"=w242, "error in (no error)"=w246, "GPIB Address"=w238) -> ("Error Out"=w244:errorcluster, "GPIB Address Out"=w245:string)  [unwired: 4 in]
                    }
                    frame #2 {
                      n71 = call "EG2001 Move Z Up.vi"("error in (no error)"=w248, "GPIB Address"=w249) -> ()  [unwired: 10 out]
                    }
                    frame #3 {
                      n72 = local read "SMU"() -> (w258:refnum<visa-resource-name>)
                      n73 = local read "Imeas Settings"() -> (w257:T10)
                      n74 = local read "Channel"() -> (w256:enum32{"Channel A", "Channel B"})
                      n75 = local read "V set"() -> (w250:dbl)
                      n76 = local read "NPLC"() -> (w255:dbl)
                      n77 = local read "I compliance"() -> (w254:dbl)
                      n78 = local read "Repeat Id"() -> (w253:u32)
                      n79 = local read "Id delay ms"() -> (w252:dbl)
                      n80 = Bundle By Name(cluster=w257, "Channel"=w256, "Vset"=w250, "NPLC"=w255, "I compliance"=w254, "Repeat time"=w253, "Delay ms"=w252) -> (w251:T10)
                      n81 = call "K2602 setVmeasI.vi"("Settings"=w251, "SMU"=w258) -> ("Iavg"=w259:dbl)  [unwired: 6 in, 3 out]
                    }
                    frame #4 {
                      n82 = local read "Vmeas Settings"() -> (w269:T9)
                      n83 = local read "Channel"() -> (w267:enum32{"Channel A", "Channel B"})
                      n84 = local read "NPLC"() -> (w261:dbl)
                      n85 = local read "V compliance"() -> (w266:dbl)
                      n86 = local read "Repeat Vf"() -> (w265:u32)
                      n87 = local read "Vf delay ms"() -> (w264:dbl)
                      n88 = local read "I set"() -> (w260:dbl)
                      n89 = Bundle By Name(cluster=w269, "Channel"=w267, "Iset"=w260, "NPLC"=w261, "V compliance"=w266, "Repeat time"=w265, "Delay ms"=w264) -> (w268:T9)
                      n90 = call "K2602 setImeasV.vi"("Settings"=w268, "SMU"=w270) -> ("Vavg"=w263:dbl)  [unwired: 6 in, 3 out]
                    }
                    frame #5 {
                      n91 = local read "I meas"() -> (w289:dbl[])
                      n92 = local read "V meas"() -> (w288:dbl[])
                      n93 = Get Date/Time In Seconds() -> (seconds since 1Jan1904=w279:timestamp)
                      n94 = Replace Array Subset(array=w289, new element=w281, index=w287) -> (w284:dbl[])
                      n95 = Replace Array Subset(array=w288, new element=w280, index=w287) -> (w283:dbl[])
                      n96 = call <vilib>:"Histogram.vi"("X"=w283) -> ("Histogram Graph"=→"Vforward hist":T13)  [unwired: 7 in, 3 out]
                      n97 = local read "Selected Data"() -> (w272:cluster{dbl[], dbl[]})
                      n98 = local write "V meas"(w283) -> ()
                      n99 = local write "I meas"(w284) -> ()
                      n100 = Bundle("V meas"=w283, "I meas"=w284) -> (w273:cluster{"V meas":dbl[], "I meas":dbl[]})  [unwired: 1 in]
                      n101 = Bundle By Name(cluster="Test Results 2", "I meas"=w281, "V meas"=w280, "Time"=w279) -> (w277:T4)
                      n102 = call <vilib>:"Histogram.vi"("X"=w284) -> ("Histogram Graph"=→"Idark hist":T13)  [unwired: 7 in, 3 out]
                      n103 = local write "Test Results"(w277) -> ()
                      n104 = local read "Session Info"() -> (w274:T5)
                      n105 = local read "Die Info"() -> (w275:T6)
                      n106 = local read "Wafer Info"() -> (w276:T7)
                      n107 = Build Array(w273, w272) -> (→"Spec Plot":cluster{"V meas":dbl[], "I meas":dbl[]}[])
                      n108 = call "writeFile RawTestData.vi"("Test Results"=w277, "Session Info"=w274, "Die Info"=w275, "Wafer Info"=w276, "Path"=w278) -> ()  [unwired: 6 in, 1 out]
                    }
                  }
                  n109 = Divide(x=w191, y=w202) -> (x/y=w200:dbl)
                  n110 = Multiply(x=w200, y=100.0) -> (x*y=w198:dbl)
                  n111 = To Unsigned Byte Integer(number=w198) -> (unsigned 8bit integer=w201:u8)
                  n112 = local write "Progress"(w201) -> ()
                  n113 = Increment(x=w191) -> (x+1=w194:i32)
                  n114 = Number To Decimal String(number=w194) -> (decimal integer string=w196:string)  [unwired: 1 in]
                  n115 = Concatenate Strings("Raw Test for die number:" ("string"), w196) -> (w197:string)
                  n116 = local write "Status"(w197) -> ()
                }
              }
              frame #3 {
                w294 = -1
                n117 = local read "TestID file"() -> (w290:path)
                n118 = local read "RawTest ID"() -> (w291:u32)
                n119 = local read "current x"() -> (w296:i32)
                n120 = local read "current y"() -> (w295:i32)
                n121 = local read "Prober GPIB"() -> (w301:string)
                n122 = call "EG2001 Move Z Down.vi"("GPIB Address"=w301) -> ("Error Out"=w300:errorcluster, "GPIB Address Out"=w299:string)  [unwired: 9 in]
                n123 = call "writeFile TestID.vi"("TestID"=w291, "Path"=w290) -> ()  [unwired: 10 in]
                n124 = Multiply(x=w294, y=w296) -> (x*y=w293:i32)
                n125 = Multiply(x=w294, y=w295) -> (x*y=w292:i32)
                n126 = call "EG2001 Move Machine Step X-Y.vi"("Flip X Coordinates?"=FALSE, "Y"=w292, "Steps/Microns"=enum32{"Steps", "Microns"}."Microns", "X"=w293, "error in (no error)"=w300, "GPIB Address"=w299) -> ()  [unwired: 4 in, 2 out]
              }
              frame #4 {
                w302 = 0
                n127 = local write "current x"(w302) -> ()
                n128 = local write "current y"(w302) -> ()
              }
            }
            n129 = Enqueue Element At Opposite End(queue=w146, element="idle", error in (no error)=w143) -> (queue out=w145:refnum<queue>, error out=w144:errorcluster)  [unwired: 1 in, 1 out]
          }
          frame "reset xy" {
            n130 = Enqueue Element At Opposite End(queue=w306, element="idle", error in (no error)=w303) -> (queue out=w305:refnum<queue>, error out=w304:errorcluster)  [unwired: 1 in, 1 out]
            "current x" <- u32 0 ("current x")
            "current y" <- u32 0 ("current y")
          }
          frame "reset to 1st die" {
            n131 = local read "Array of Cell Data Clusters"() -> (w320:T11)
            n132 = Index Array(array=w320, index=0) -> (element=w318:T14)
            n133 = Unbundle By Name(w318) -> ("X-coord"=w317:dbl, "Y-coord"=w316:dbl)
            n134 = local write "current x"(w317) -> ()
            n135 = local write "current y"(w316) -> ()
            n136 = Enqueue Element At Opposite End(queue=w313, element="idle", error in (no error)=w314) -> (queue out=w312:refnum<queue>, error out=w311:errorcluster)  [unwired: 1 in, 1 out]
          }
          frame "load file manual" {
            n137 = flat-sequence {
              tunnel: [w332] -> w327
              tunnel: w327 -> [w336]
              frame #0 {
                n138 = call "Device Files v1.vi"("Rows"=1200, "Mask file path"="Mask File Manual") -> ("Mask Name"=w333:string, "size(s)"=w332:i32, "Array of Cell Clusters"=w329:T3)  [unwired: 6 in, 1 out]
                n139 = local write "Array of Cell Data Clusters"(w329) -> ()
                n140 = local write "Status"("Loading mask file" ("Status")) -> ()
                n141 = local write "Mask"(w333) -> ()
              }
              frame #1 {
                n142 = for {
                  N: w336 -> [_]
                  tunnel: [w337] -> w335 mode=indexing
                  i -> [w338]
                  n143 = Number To Decimal String(number=w338) -> (decimal integer string=w337:string)  [unwired: 1 in]
                }
                n144 = property on="Die Number" class="Ring (strict)"("Strings []"=w335) -> ()  [unwired: 2 in, 2 out]
              }
              frame #2 {
                n145 = local read "Array of Cell Data Clusters"() -> (w346:T11)
                n146 = local read "Die Number"() -> (w345:u16)
                n147 = Index Array(array=w346, index=w345) -> (element=w344:T14)
                n148 = Unbundle By Name(w344) -> ("Cell Name"=w339:string, "X-coord"=w342:dbl, "Y-coord"=w343:dbl, "Area"=w341:dbl, "Meas Area"=w340:dbl)
                n149 = local write "Device Name"(w339) -> ()
                n150 = local write "x target"(w342) -> ()
                n151 = local write "y target"(w343) -> ()
                n152 = local write "ActiveArea_um2"(w341) -> ()
                n153 = local write "MesaArea_um2"(w340) -> ()
              }
              frame #3 {
                n154 = local read "Laser Power (mW)"() -> (w349:dbl)
                n155 = Equal To 0?(x=w349) -> (x = 0?=w348:bool)
                n156 = case shown="True" w348 {
                  tunnel: [w354 w355] -> w347
                  frame False {
                    n157 = local read "ActiveArea_um2"() -> (w354:dbl)
                  }
                  frame True {
                    n158 = local read "MesaArea_um2"() -> (w355:dbl)
                  }
                }
                n159 = local read "J set A/cm2"() -> (w352:dbl)
                n160 = Divide(x=w347, y=100000000.0) -> (x/y=w351:dbl)
                n161 = Multiply(x=w351, y=w352) -> (x*y=w353:dbl)
                n162 = local write "I set"(w353) -> ()
              }
            }
            n163 = Enqueue Element At Opposite End(queue=w324, element="idle", error in (no error)=w325) -> (queue out=w323:refnum<queue>, error out=w322:errorcluster)  [unwired: 1 in, 1 out]
          }
          frame "Die number picked" {
            n164 = flat-sequence {
              frame #0 {
                n165 = local read "Array of Cell Data Clusters"() -> (w370:T11)
                n166 = local read "Die Number"() -> (w369:u16)
                n167 = Index Array(array=w370, index=w369) -> (element=w368:T14)
                n168 = Unbundle By Name(w368) -> ("Cell Name"=w365:string, "X-coord"=w367:dbl, "Y-coord"=w366:dbl, "Area"=w364:dbl, "Meas Area"=w363:dbl)
                n169 = local write "Device Name"(w365) -> ()
                n170 = local write "x target"(w367) -> ()
                n171 = local write "y target"(w366) -> ()
                n172 = local write "ActiveArea_um2"(w364) -> ()
                n173 = local write "MesaArea_um2"(w363) -> ()
              }
              frame #1 {
                n174 = local read "Laser Power (mW)"() -> (w373:dbl)
                n175 = Equal To 0?(x=w373) -> (x = 0?=w372:bool)
                n176 = case shown="True" w372 {
                  tunnel: [w378 w379] -> w371
                  frame False {
                    n177 = local read "ActiveArea_um2"() -> (w378:dbl)
                  }
                  frame True {
                    n178 = local read "MesaArea_um2"() -> (w379:dbl)
                  }
                }
                n179 = local read "J set A/cm2"() -> (w376:dbl)
                n180 = Divide(x=w371, y=100000000.0) -> (x/y=w375:dbl)
                n181 = Multiply(x=w375, y=w376) -> (x*y=w377:dbl)
                n182 = local write "I set"(w377) -> ()
              }
            }
            n183 = local write "Status"("Changing Die" ("Status")) -> ()
            n184 = Enqueue Element At Opposite End(queue=w357, element="idle", error in (no error)=w356) -> (queue out=w358:refnum<queue>, error out=w359:errorcluster)  [unwired: 1 in, 1 out]
          }
          frame "Jset change" {
            n185 = local read "ActiveArea_um2"() -> (w389:dbl)
            n186 = local read "J set A/cm2"() -> (w386:dbl)
            n187 = Divide(x=w389, y=100000000.0) -> (x/y=w387:dbl)
            n188 = Multiply(x=w387, y=w386) -> (x*y=w385:dbl)
            n189 = local write "I set"(w385) -> ()
            n190 = Enqueue Element At Opposite End(queue=w383, element="idle", error in (no error)=w380) -> (queue out=w382:refnum<queue>, error out=w381:errorcluster)  [unwired: 1 in, 1 out]
          }
          frame "moveto" {
            n191 = flat-sequence {
              tunnel: [w402] -> w395
              tunnel: [w401] -> w394
              tunnel: w395 -> [w411]
              tunnel: w394 -> [w410]
              tunnel: [w406] -> w392
              tunnel: [w405] -> w391
              tunnel: w392 -> [w419]
              tunnel: w391 -> [w418]
              frame #0 {
                n192 = local read "Prober GPIB"() -> (w403:string)
                n193 = local write "Status"("Probe up" ("Status")) -> ()
                n194 = call "EG2001 Move Z Down.vi"("GPIB Address"=w403) -> ("Error Out"=w401:errorcluster, "GPIB Address Out"=w402:string)  [unwired: 9 in]
              }
              frame #1 {
                n195 = local read "y target"() -> (w415:i32)
                n196 = local read "x target"() -> (w417:i32)
                n197 = local read "current x"() -> (w416:i32)
                n198 = local read "current y"() -> (w414:i32)
                n199 = local write "Status"("Moving Probe" ("Status")) -> ()
                n200 = Subtract(x=w417, y=w416) -> (x-y=w413:i32)
                n201 = Subtract(x=w415, y=w414) -> (x-y=w412:i32)
                n202 = call "EG2001 Move Machine Step X-Y.vi"("Flip X Coordinates?"=FALSE, "Y"=w412, "Steps/Microns"=enum32{"Steps", "Microns"}."Microns", "X"=w413, "error in (no error)"=w410, "GPIB Address"=w411) -> ("Error Out"=w405:errorcluster, "GPIB Address Out"=w406:string)  [unwired: 4 in]
              }
              frame #2 {
                n203 = local read "x target"() -> (w422:i32)
                n204 = local read "y target"() -> (w421:i32)
                n205 = call "EG2001 Move Z Up.vi"("error in (no error)"=w418, "GPIB Address"=w419) -> ()  [unwired: 8 in, 2 out]
                n206 = local write "current y"(w421) -> ()
                n207 = local write "current x"(w422) -> ()
                n208 = local write "Status"("Done" ("Status")) -> ()
              }
            }
            n209 = Enqueue Element At Opposite End(queue=w398, element="idle", error in (no error)=w393) -> (queue out=w397:refnum<queue>, error out=w396:errorcluster)  [unwired: 1 in, 1 out]
          }
          frame "movetofirst" {
            n210 = flat-sequence {
              tunnel: [w436] -> w427
              tunnel: [w435] -> w426
              tunnel: w427 -> [w441]
              tunnel: w426 -> [w440]
              tunnel: [w438] -> w424
              tunnel: [w437] -> w423
              tunnel: w424 -> [w444]
              tunnel: w423 -> [w443]
              frame #0 {
                n211 = local read "Prober GPIB"() -> (w434:string)
                n212 = local write "Status"("Probe up" ("Status")) -> ()
                n213 = call "EG2001 Move Z Down.vi"("GPIB Address"=w434) -> ("Error Out"=w435:errorcluster, "GPIB Address Out"=w436:string)  [unwired: 9 in]
              }
              frame #1 {
                n214 = local write "Status"("Moving Probe" ("Status")) -> ()
                n215 = call "EG2001 Move First.vi"("error in (no error)"=w440, "GPIB Address"=w441) -> ("Error Out"=w437:errorcluster, "GPIB Address Out"=w438:string)  [unwired: 8 in]
              }
              frame #2 {
                w442 = 0 ("current x")
                n216 = call "EG2001 Move Z Up.vi"("error in (no error)"=w443, "GPIB Address"=w444) -> ()  [unwired: 8 in, 2 out]
                n217 = local write "current y"(w442) -> ()
                n218 = local write "current x"(w442) -> ()
                n219 = local write "Status"("Done" ("Status")) -> ()
              }
            }
            n220 = Enqueue Element At Opposite End(queue=w430, element="idle", error in (no error)=w425) -> (queue out=w429:refnum<queue>, error out=w428:errorcluster)  [unwired: 1 in, 1 out]
          }
          frame "manual test" {
            n221 = flat-sequence {
              tunnel: [w463] -> w460
              tunnel: [w462] -> w459
              tunnel: [w468] -> w458
              tunnel: [w467] -> w457
              tunnel: w460 -> [w467]
              tunnel: [w466] -> w456
              tunnel: w459 -> [w466]
              tunnel: w458 -> [w492]
              tunnel: [w492] -> w455
              tunnel: [w482] -> w454
              tunnel: w457 -> [w482]
              tunnel: [w481] -> w453
              tunnel: w456 -> [w481]
              tunnel: w455 -> [w505]
              tunnel: [w495] -> w452
              tunnel: w454 -> [w495]
              tunnel: [w494] -> w451
              tunnel: w453 -> [w494]
              tunnel: w452 -> [w519]
              tunnel: w451 -> [w518]
              frame #0 {
                n222 = local read "Prober GPIB"() -> (w464:string)
                n223 = call "EG2001 Move Z Up.vi"("GPIB Address"=w464) -> ("Error Out"=w462:errorcluster, "GPIB Address Out"=w463:string)  [unwired: 1 in, 8 out]
              }
              frame #1 {
                n224 = local read "SMU"() -> (w468:refnum<visa-resource-name>)
                n225 = local read "Sweep Settings"() -> (w479:T8)
                n226 = local read "Channel"() -> (w478:enum32{"Channel A", "Channel B"})
                n227 = local read "V start"() -> (w477:dbl)
                n228 = local read "V end"() -> (w476:dbl)
                n229 = local read "points"() -> (w475:u16)
                n230 = local read "NPLC"() -> (w474:dbl)
                n231 = local read "I compliance"() -> (w473:dbl)
                n232 = local read "sweep delay ms"() -> (w472:dbl)
                n233 = Bundle By Name(cluster=w479, "Channel"=w478, "Vstart"=w477, "Vend"=w476, "# of points"=w475, "NPLC"=w474, "I compliance"=w473, "Delay ms"=w472) -> (w471:T8)
                n234 = call "K2602 Vsweep.vi"("Settings"=w471, "SMU"=w468) -> ("V"=→"Varray manual":dbl[], "I"=→"Iarray manual":dbl[])  [unwired: 7 in, 1 out]
                n235 = local write "Status"("Sweeping IV Curve") -> ()
              }
              frame #2 {
                n236 = local read "Imeas Settings"() -> (w491:T10)
                n237 = local read "Channel"() -> (w488:enum32{"Channel A", "Channel B"})
                n238 = local read "V set"() -> (w487:dbl)
                n239 = local read "NPLC"() -> (w486:dbl)
                n240 = local read "I compliance"() -> (w485:dbl)
                n241 = local read "Repeat Id"() -> (w484:u32)
                n242 = local read "Id delay ms"() -> (w483:dbl)
                n243 = Bundle By Name(cluster=w491, "Channel"=w488, "Vset"=w487, "NPLC"=w486, "I compliance"=w485, "Repeat time"=w484, "Delay ms"=w483) -> (w490:T10)
                n244 = local write "Status"("Measuring I @ Vset") -> ()
                n245 = call "K2602 setVmeasI.vi"("Settings"=w490, "SMU"=w492) -> ("Iavg"=w489:dbl)  [unwired: 6 in, 3 out]
                n246 = local write "Imeas manual"(w489) -> ()
              }
              frame #3 {
                n247 = local read "Vmeas Settings"() -> (w503:T9)
                n248 = local read "Channel"() -> (w501:enum32{"Channel A", "Channel B"})
                n249 = local read "I set"() -> (w500:dbl)
                n250 = local read "NPLC"() -> (w499:dbl)
                n251 = local read "V compliance"() -> (w498:dbl)
                n252 = local read "Repeat Vf"() -> (w497:u32)
                n253 = local read "Vf delay ms"() -> (w496:dbl)
                n254 = Bundle By Name(cluster=w503, "Channel"=w501, "Iset"=w500, "NPLC"=w499, "V compliance"=w498, "Repeat time"=w497, "Delay ms"=w496) -> (w502:T9)
                n255 = local write "Status"("Measuring V @ Iset") -> ()
                n256 = call "K2602 setImeasV.vi"("Settings"=w502, "SMU"=w505) -> ("Vavg"=w504:dbl)  [unwired: 6 in, 3 out]
                n257 = local write "Vmeas manual"(w504) -> ()
              }
              frame #4 {
                n258 = local read "Imeas manual"() -> (w508:dbl)
                n259 = local read "Vmeas manual"() -> (w509:dbl)
                n260 = local read "points"() -> (w512:u16)
                n261 = local read "Varray manual"() -> (w511:dbl[])
                n262 = local read "Iarray manual"() -> (w510:dbl[])
                n263 = local read "V set"() -> (w507:dbl)
                n264 = local read "I set"() -> (w506:dbl)
                n265 = call "EG2001 Move Z Down.vi"("error in (no error)"=w518, "GPIB Address"=w519) -> ()  [unwired: 8 in, 2 out]
                n266 = local write "Status"("Done") -> ()
                n267 = local read "Manual IV settting"() -> (w517:enum32{"Linear plot", "Log plot"})
                n268 = call "get Plot.vi"("I set"=w506, "Imeas"=w508, "V set"=w507, "Vmeas"=w509, "Iarray"=w510, "Varray"=w511, "points"=w512) -> ("logplot"=w514:cluster{"Varray manual":dbl[], dbl[]}[], "Linearplot"=w513:T15)  [unwired: 3 in]
                "Manual Plot 0" <- w513
                "Manaul Plot 1" <- w514
                n269 = case shown="\"Linear plot\", Default" w517 {
                  tunnel: w513 -> [w522 _]
                  tunnel: [w522 w525] -> w516
                  tunnel: w514 -> [_ w525]
                  frame "Linear plot", Default {
                    n270 = property on="Manual IV" class="XYGraph (strict)"("YScale.Mapping Mode"=u8 0 ("Y Scale.Mapping Mode")) -> ()  [unwired: 2 in, 2 out]
                    n271 = property on="Manual IV" class="XYGraph (strict)"("YScale.NameLbl.Text"="Current (A)" ("X Scale.Name Label.Text")) -> ()  [unwired: 2 in, 2 out]
                  }
                  frame "Log plot" {
                    n272 = property on="Manual IV" class="XYGraph (strict)"("YScale.NameLbl.Text"="Abs(I)" ("Y Scale.Name Label.Text")) -> ()  [unwired: 2 in, 2 out]
                    n273 = property on="Manual IV" class="XYGraph (strict)"("YScale.Mapping Mode"=u8 1 ("Y Scale.Mapping Mode")) -> ()  [unwired: 2 in, 2 out]
                  }
                }
                "Manual IV" <- w516
              }
            }
            n274 = Enqueue Element At Opposite End(queue=w447, element="idle", error in (no error)=w450) -> (queue out=w448:refnum<queue>, error out=w449:errorcluster)  [unwired: 1 in, 1 out]
          }
          frame "update wafer" {
            n275 = local read "Wafer Name"() -> (w528:string)
            n276 = call "getDB Wafer Info.vi"("Wafer Name"=w528) -> ("WaferInfo"=w529:T16)  [unwired: 9 in, 1 out]
            n277 = Unbundle By Name(w529) -> ("WaferName"=w526:string, "Scribe"=w534:string, "Lot"=w533:string, "Mask"=w532:string)  [unwired: 1 out]
            n278 = local write "Scribe"(w534) -> ()
            n279 = local write "Lot"(w533) -> ()
            n280 = local write "Mask"(w532) -> ()
            n281 = Equal?(x=w528, y=w526) -> (x = y?=w527:bool)
            n282 = case shown="False" w527 {
              tunnel: w526 -> [w539 _]
              frame False {
                n283 = local write "Wafer Name"(w539) -> ()
              }
              frame True {
              }
            }
            n284 = Enqueue Element At Opposite End(queue=w537, element="idle", error in (no error)=w530) -> (queue out=w536:refnum<queue>, error out=w535:errorcluster)  [unwired: 1 in, 1 out]
          }
          frame "idle" {
            n285 = local write "Status"("idle" ("Status")) -> ()
          }
          frame "change plot" {
            n286 = local read "Manual IV settting"() -> (w551:enum32{"Linear plot", "Log plot"})
            n287 = case shown="\"Log plot\"" w551 {
              tunnel: [w554 w557] -> w550
              frame "Linear plot", Default {
                n288 = local read "Manual Plot 0"() -> (w554:cluster{"V manual":dbl[], "I manual":dbl[]}[])
                n289 = property on="Manual IV" class="XYGraph (strict)"("YScale.NameLbl.Text"="Current (A)" ("Y Scale.Name Label.Text")) -> ()  [unwired: 2 in, 2 out]
                n290 = property on="Manual IV" class="XYGraph (strict)"("YScale.Mapping Mode"=u8 0 ("Y Scale.Mapping Mode")) -> ()  [unwired: 2 in, 2 out]
              }
              frame "Log plot" {
                n291 = local read "Manaul Plot 1"() -> (w557:cluster{"V manual":dbl[], dbl[]}[])
                n292 = property on="Manual IV" class="XYGraph (strict)"("YScale.Mapping Mode"=u8 1 ("Y Scale.Mapping Mode")) -> ()  [unwired: 2 in, 2 out]
                n293 = property on="Manual IV" class="XYGraph (strict)"("YScale.NameLbl.Text"="Abs(I)" ("Y Scale.Name Label.Text")) -> ()  [unwired: 2 in, 2 out]
              }
            }
            n294 = local write "Manual IV"(w550) -> ()
            n295 = Enqueue Element At Opposite End(queue=w545, element="idle", error in (no error)=w547) -> (queue out=w544:refnum<queue>, error out=w546:errorcluster)  [unwired: 1 in, 1 out]
          }
          frame "select" {
            n296 = local read "I meas"() -> (w560:dbl[])
            n297 = Array Size(array=w560) -> (size(s)=w558:i32)
            n298 = Greater Than 0?(x=w558) -> (x > 0?=w559:bool)
            n299 = case shown="True" w559 {
              tunnel: w558 -> [_ w582]
              frame False {
              }
              frame True {
                n300 = local read "Number Select"() -> (w588:u16)
                n301 = local read "I meas"() -> (w573:dbl[])
                n302 = local read "V meas"() -> (w574:dbl[])
                n303 = local read "Vmin"() -> (w586:dbl)
                n304 = local read "Vmax"() -> (w587:dbl)
                n305 = local read "RawData Save Path"() -> (w584:path)
                n306 = local read "Mask File Raw"() -> (w589:path)
                n307 = local read "Wafer Name"() -> (w590:string)
                n308 = Initialize Array(nan ("element"), w582) -> (w578:dbl[])
                n309 = call "select RawTestData.vi"("Number Select"=w588, "Vmax"=w587, "Vmin"=w586, "V meas"=w574, "I meas"=w573) -> ("Selected V"=w581:dbl[], "Selected I"=w579:dbl[], "Selected Index"=w567:dbl[])  [unwired: 3 in, 1 out]
                n310 = Replace Array Subset(array=w578, new element=w581, index=0) -> (w576:dbl[])
                n311 = Replace Array Subset(array=w578, new element=w579, index=0) -> (w575:dbl[])
                n312 = call "save FineMask.vi"("Selected Index"=w567, "RawData Save Path"=w584, "Text Add"=w590, "Mask File Raw"=w589) -> ("Output path"=w585:path)  [unwired: 7 in]
                n313 = local read "RawData file"() -> (w569:path)
                n314 = Bundle(w576, w575) -> (w571:cluster{dbl[], dbl[]})  [unwired: 1 in]
                n315 = Bundle("V meas"=w574, "I meas"=w573) -> (w572:cluster{"V meas":dbl[], "I meas":dbl[]})  [unwired: 1 in]
                n316 = local write "Mask File Fine"(w585) -> ()
                n317 = Build Array(w572, w571) -> (w570:cluster{"V meas":dbl[], "I meas":dbl[]}[])
                n318 = call "updatedFile RawTestSelect.vi"("Column Number"=u32 21, "Selected Index"=w567, "Path"=w569) -> ()  [unwired: 9 in]
                n319 = local write "Spec Plot"(w570) -> ()
              }
            }
            n320 = Enqueue Element At Opposite End(queue=w563, element="idle", error in (no error)=w562) -> (queue out=w565:refnum<queue>, error out=w564:errorcluster)  [unwired: 1 in, 1 out]
          }
          frame "load raw data" {
            n321 = local read "RawData Save Path"() -> (w593:path)
            n322 = call "File Dialog"("start path"=w593, "prompt"="Please pick a raw test data file", "pattern (all files)"="*.csv" ("pattern label")) -> ("selected path"=w592:path, "cancelled"=w596:bool)  [unwired: 9 in, 2 out]
            n323 = case shown="False" w596 {
              tunnel: w592 -> [_ w602]
              frame True {
              }
              frame False {
                n324 = call "read Raw.vi"("Path"=w602) -> ("Session Info"=w621:T17, "Die Info"=w630:T18, "Wafer Info"=w629:T7, "V"=w607:dbl[], "I"=w606:dbl[])  [unwired: 6 in]
                n325 = Array Size(array=w606) -> (size(s)=w612:i32)
                n326 = Strip Path(path=w602) -> (name=w603:string)  [unwired: 1 out]
                n327 = local write "V meas"(w607) -> ()
                n328 = local write "I meas"(w606) -> ()
                n329 = Initialize Array(nan ("element"), w612) -> (w611:dbl[])
                n330 = Unbundle By Name(w629) -> ("Wafer Name"=w628:string, "Scribe"=w627:string, "Mask"=w626:string, "Lot"=w625:string)
                n331 = local write "RawData file"(w602) -> ()
                n332 = Bundle("V"=w607, "I"=w606) -> (w610:cluster{"V":dbl[], "I":dbl[]})  [unwired: 1 in]
                n333 = Bundle(w611, w611) -> (w609:cluster{dbl[], dbl[]})  [unwired: 1 in]
                n334 = local write "Test FileName"(w603) -> ()
                n335 = local write "Wafer Name"(w628) -> ()
                n336 = local write "Scribe"(w627) -> ()
                n337 = local write "Mask"(w626) -> ()
                n338 = local write "Lot"(w625) -> ()
                n339 = local write "Selected Data"(w609) -> ()
                n340 = call <vilib>:"Histogram.vi"("X"=w606) -> ("Histogram Graph"=w605:T13)  [unwired: 7 in, 3 out]
                n341 = call <vilib>:"Histogram.vi"("X"=w607) -> ("Histogram Graph"=w604:T13)  [unwired: 7 in, 3 out]
                n342 = Build Array(w610, w609) -> (w608:cluster{"V":dbl[], "I":dbl[]}[])
                n343 = Unbundle By Name(w630) -> ("Device Name"=w624:string, "ActiveArea_um2"=w623:dbl, "MesaArea_um2"=w622:dbl)
                n344 = local write "Vforward hist"(w604) -> ()
                n345 = local write "Idark hist"(w605) -> ()
                n346 = local write "Spec Plot"(w608) -> ()
                n347 = local write "Device Name"(w624) -> ()
                n348 = local write "ActiveArea_um2"(w623) -> ()
                n349 = local write "MesaArea_um2"(w622) -> ()
                n350 = Unbundle By Name(w621) -> ("V set"=w620:dbl, "I compliance"=w619:dbl, "J set"=w618:dbl, "I set"=w617:dbl, "V compliance"=w616:dbl, "Laser Power (mW)"=w614:dbl, "Operator"=w615:string)
                n351 = local write "V set"(w620) -> ()
                n352 = local write "I compliance"(w619) -> ()
                n353 = local write "J set A/cm2"(w618) -> ()
                n354 = local write "I set"(w617) -> ()
                n355 = local write "V compliance"(w616) -> ()
                n356 = local write "Laser Power (mW)"(w614) -> ()
                n357 = local write "Operator"(w615) -> ()
              }
            }
            n358 = Enqueue Element At Opposite End(queue=w598, element="idle", error in (no error)=w597) -> (queue out=w600:refnum<queue>, error out=w599:errorcluster)  [unwired: 1 in, 1 out]
          }
          frame "start fine" {
            n359 = flat-sequence {
              tunnel: [w638] -> w632
              tunnel: w632 -> [w649]
              frame #0 {
                w639 = u8 0 ("Progress 2")
                n360 = local read "points"() -> (w641:u16)
                n361 = Initialize Array(nan ("element"), w641) -> (w643:dbl[])
                n362 = Bundle(w643, w643) -> (w642:cluster{dbl[], dbl[]})  [unwired: 1 in]
                n363 = call "Device Files v1.vi"("Rows"=1200, "Mask file path"="Mask File Fine") -> ("size(s)"=w638:i32, "Array of Cell Clusters"=→"Fine Cell Clusters":T3)  [unwired: 6 in, 2 out]
                "Total Device" <- w638
                n364 = local write "Status"("prepare fine test" ("Status")) -> ()
                n365 = local write "Progress 2"(w639) -> ()
                n366 = Initialize Array(w642, w638) -> (→"IV fine linear" →"IV fine log":cluster{dbl[], dbl[]}[])
                "Current Device" <- w639
              }
              frame #1 {
                n367 = for {
                  N: w649 -> [w673]
                  i -> [w674]
                  n368 = Increment(x=w674) -> (x+1=w653:i32)
                  n369 = flat-sequence {
                    tunnel: w674 -> [w680]
                    tunnel: [w688] -> w668
                    tunnel: [w687] -> w667
                    tunnel: [w684] -> w666
                    tunnel: [w683] -> w665
                    tunnel: [w682] -> w664
                    tunnel: [w681] -> w663
                    tunnel: [w680] -> w654
                    tunnel: w668 -> [w703]
                    tunnel: w667 -> [w702]
                    tunnel: w666 -> [w700]
                    tunnel: w665 -> [w699]
                    tunnel: w664 -> [w698]
                    tunnel: w663 -> [w697]
                    tunnel: [w696] -> w662
                    tunnel: [w695] -> w661
                    tunnel: [w694] -> w655
                    tunnel: w654 -> [w694]
                    tunnel: w662 -> [w706]
                    tunnel: w661 -> [w705]
                    tunnel: [w704] -> w656
                    tunnel: w655 -> [w704]
                    tunnel: [w710] -> w657
                    tunnel: w656 -> [w710]
                    tunnel: w657 -> [w740]
                    tunnel: [w730] -> w652
                    tunnel: [w724] -> w651
                    tunnel: [w723] -> w650
                    tunnel: w652 -> [w757]
                    tunnel: w651 -> [w750]
                    tunnel: w650 -> [w749]
                    frame #0 {
                      n370 = local read "Fine Cell Clusters"() -> (w693:T3)
                      n371 = local read "Laser Power (mW)"() -> (w676:dbl)
                      n372 = local read "Prober GPIB"() -> (w689:string)
                      n373 = Index Array(array=w693, index=w680) -> (element=w677:T19)
                      n374 = Unbundle By Name(w677) -> ("Cell Name"=w692:string, "X-coord"=w682:dbl, "Y-coord"=w681:dbl, "Area"=w691:dbl, "Mesa Area"=w690:dbl)
                      n375 = local read "current x"() -> (w686:i32)
                      n376 = local read "current y"() -> (w685:i32)
                      n377 = call "get Area.vi"("Laser"=w676, "Cell Data Cluster"=w677) -> ("Area"=w678:dbl)  [unwired: 9 in]
                      n378 = local read "Parameters Flash 2"() -> (w679:T2)
                      n379 = Bundle By Name(cluster=w679, "Cell Area (cm²)"=w678) -> (w675:T2)
                      n380 = call "EG2001 Move Z Down.vi"("GPIB Address"=w689) -> ("Error Out"=w687:errorcluster, "GPIB Address Out"=w688:string)  [unwired: 9 in]
                      n381 = local write "Parameters Flash"(w675) -> ()
                      n382 = Subtract(x=w682, y=w686) -> (x-y=w684:dbl)
                      n383 = Subtract(x=w681, y=w685) -> (x-y=w683:dbl)
                      n384 = local write "Device Name"(w692) -> ()
                      n385 = local write "ActiveArea_um2"(w691) -> ()
                      n386 = local write "MesaArea_um2"(w690) -> ()
                    }
                    frame #1 {
                      n387 = local write "current x"(w698) -> ()
                      n388 = local write "current y"(w697) -> ()
                      n389 = call "EG2001 Move Machine Step X-Y.vi"("Y"=w699, "Steps/Microns"=enum32{"Steps", "Microns"}."Microns", "X"=w700, "error in (no error)"=w702, "GPIB Address"=w703) -> ("Error Out"=w695:errorcluster, "GPIB Address Out"=w696:string)  [unwired: 5 in]
                    }
                    frame #2 {
                      n390 = call "EG2001 Move Z Up.vi"("error in (no error)"=w705, "GPIB Address"=w706) -> ()  [unwired: 10 out]
                    }
                    frame #3 {
                      n391 = local read "SMU"() -> (w722:refnum<visa-resource-name>)
                      n392 = local read "Sweep Settings"() -> (w721:T8)
                      n393 = local read "Channel"() -> (w719:enum32{"Channel A", "Channel B"})
                      n394 = local read "V start"() -> (w717:dbl)
                      n395 = local read "V end"() -> (w718:dbl)
                      n396 = local read "points"() -> (w716:u16)
                      n397 = local read "NPLC"() -> (w715:dbl)
                      n398 = local read "I compliance"() -> (w714:dbl)
                      n399 = local read "sweep delay ms"() -> (w713:dbl)
                      n400 = local read "Device Name"() -> (w708:string)
                      n401 = local read "Wafer Info Flash 2"() -> (w709:T1)
                      n402 = Bundle By Name(cluster=w709, "Cell Name"=w708) -> (w707:T1)
                      n403 = local write "Wafer Info Flash"(w707) -> ()
                      n404 = Bundle By Name(cluster=w721, "Channel"=w719, "Vstart"=w717, "Vend"=w718, "# of points"=w716, "NPLC"=w715, "I compliance"=w714, "Delay ms"=w713) -> (w720:T8)
                      n405 = call "K2602 Vsweep.vi"("Settings"=w720, "SMU"=w722) -> ("V"=w711:dbl[], "I"=w712:dbl[])  [unwired: 7 in, 1 out]
                      n406 = local write "I fine"(w712) -> ()
                      n407 = local write "V fine"(w711) -> ()
                    }
                    frame #4 {
                      n408 = local read "V fine"() -> (w729:dbl[])
                      n409 = local read "I fine"() -> (w736:dbl[])
                      n410 = local read "IV fine linear"() -> (w743:cluster{dbl[], dbl[]}[])
                      n411 = local read "IV fine log"() -> (w738:cluster{dbl[], dbl[]}[])
                      n412 = local read "Wafer Name"() -> (w733:string)
                      n413 = local read "Operator"() -> (w732:string)
                      n414 = local read "Device Name"() -> (w731:string)
                      n415 = Get Date/Time In Seconds() -> (seconds since 1Jan1904=w723:timestamp)
                      n416 = local read "current x"() -> (w726:i32)
                      n417 = local read "current y"() -> (w725:i32)
                      n418 = Absolute Value(x=w736) -> (abs(x)=w737:dbl[])
                      n419 = Bundle("V fine"=w729, "I fine"=w736) -> (w741:cluster{"V fine":dbl[], "I fine":dbl[]})  [unwired: 1 in]
                      n420 = To Double Precision Float(number=w726) -> (double precision float=w728:dbl)
                      n421 = To Double Precision Float(number=w725) -> (double precision float=w727:dbl)
                      n422 = Bundle("V fine"=w729, w737) -> (w735:cluster{"V fine":dbl[], dbl[]})  [unwired: 1 in]
                      n423 = Replace Array Subset(array=w738, new element=w735, index=w740) -> (w739:cluster{dbl[], dbl[]}[])
                      n424 = local write "IV fine log"(w739) -> ()
                      n425 = Replace Array Subset(array=w743, new element=w741, index=w740) -> (w742:cluster{dbl[], dbl[]}[])
                      n426 = local write "IV fine linear"(w742) -> ()
                      n427 = Bundle(w728, w727) -> (w724:cluster{dbl, dbl})  [unwired: 1 in]
                      n428 = call "get Flash FileName .vi"("Time"=w723, "Device Name"=w731, "Operator"=w732, "Wafer Name"=w733, "FineTest save path"="FineTest save path") -> ("appended path"=w730:path)  [unwired: 6 in]
                    }
                    frame #5 {
                      # "Change it !!!!!!!!"
                      n429 = local read "Parameters Flash"() -> (w752:T2)
                      n430 = local read "Wafer Info Flash"() -> (w751:T1)
                      n431 = local read "I fine"() -> (w755:dbl[])
                      n432 = local read "V fine"() -> (w754:dbl[])
                      n433 = local read "Mask"() -> (w756:string)
                      n434 = Get Date/Time String(seconds (now)=w749, want seconds? (F)=TRUE) -> (date string=w748:string, time string=w745:string)  [unwired: 1 in]
                      n435 = call <vilib>:"Space Constant.vi"() -> ("String"=w744:string)
                      n436 = Concatenate Strings(w748, w744, w745) -> (w746:string)
                      n437 = Build Array(w755, w754) -> (w753:dbl[][])
                      n438 = call "WriteFlashFile.vi"("file path (dialog if empty)"=w757, "Mask Name"=w756, "IV array"=w753, "Date/Time String"=w746, "Parameters"=w752, "Coords"=w750, "Wafer Info"=w751) -> ()  [unwired: 8 in, 1 out]
                    }
                  }
                  n439 = Divide(x=w653, y=w673) -> (x/y=w672:dbl)
                  n440 = Multiply(x=100.0, y=w672) -> (x*y=w670:dbl)
                  n441 = To Unsigned Byte Integer(number=w670) -> (unsigned 8bit integer=w669:u8)
                  n442 = local write "Progress 2"(w669) -> ()
                  n443 = local write "Current Device"(w653) -> ()
                  n444 = Number To Decimal String(number=w653) -> (decimal integer string=w659:string)  [unwired: 1 in]
                  n445 = Concatenate Strings("IV test for die number: " ("string"), w659) -> (w658:string)
                  n446 = local write "Status"(w658) -> ()
                }
              }
              frame #2 {
                w762 = -1 ("x")
                n447 = local read "current x"() -> (w764:i32)
                n448 = local read "current y"() -> (w763:i32)
                n449 = local read "Prober GPIB"() -> (w766:string)
                n450 = call "EG2001 Move Z Down.vi"("GPIB Address"=w766) -> ("Error Out"=w765:errorcluster, "GPIB Address Out"=w767:string)  [unwired: 9 in]
                n451 = Multiply(x=w762, y=w764) -> (x*y=w761:i32)
                n452 = Multiply(x=w763, y=w762) -> (x*y=w760:i32)
                n453 = call "EG2001 Move Machine Step X-Y.vi"("Flip X Coordinates?"=FALSE, "Y"=w760, "Steps/Microns"=enum32{"Steps", "Microns"}."Microns", "X"=w761, "error in (no error)"=w765, "GPIB Address"=w767) -> ()  [unwired: 4 in, 2 out]
              }
              frame #3 {
                w768 = 0 ("current x")
                n454 = local write "current x"(w768) -> ()
                n455 = local write "current y"(w768) -> ()
              }
            }
            n456 = Enqueue Element At Opposite End(queue=w635, element="idle", error in (no error)=w634) -> (queue out=w637:refnum<queue>, error out=w636:errorcluster)  [unwired: 1 in, 1 out]
          }
          frame "raw mask updated" {
            n457 = Two Button Dialog(message="Wold you like to update the Manual mask?", 1:"No" ("F button name (\"Cancel\")"), 2:"Yes" ("T button name (\"OK\")")) -> (T button?=w769:bool)
            n458 = case shown="True" w769 {
              frame False {
              }
              frame True {
                n459 = local read "Mask File Raw"() -> (w779:path)
                n460 = local write "Mask File Manual"(w779) -> ()
              }
            }
            n461 = Enqueue Element At Opposite End(queue=w776, element="idle", error in (no error)=w775) -> (queue out=w778:refnum<queue>, error out=w777:errorcluster)  [unwired: 1 in, 1 out]
          }
          frame "mask manual update" {
            n462 = Two Button Dialog(message="Would you like update mask file for raw test?", 1:"No" ("F button name (\"Cancel\")"), 2:"Yes" ("T button name (\"OK\")")) -> (T button?=w780:bool)
            n463 = case shown="True" w780 {
              frame False {
              }
              frame True {
                n464 = local read "Mask File Manual"() -> (w790:path)
                n465 = local write "Mask File Raw"(w790) -> ()
              }
            }
            n466 = Enqueue Element At Opposite End(queue=w787, element="idle", error in (no error)=w786) -> (queue out=w789:refnum<queue>, error out=w788:errorcluster)  [unwired: 1 in, 1 out]
          }
        }
      }
      n467 = while {
        shift-right: [w21] -> w17
        shift-left: w16 -> [w22]
        shift-right: [w19] -> w8
        shift-left: w15 -> [w20]
        stop <- w23 stop-if-true
        n468 = event shown="[6] \"Move to 0 0\": Value Change" {
          selector: _ -> [_ _ _ _ _ _ _ _ _ _ _ _ _ _ _ _ _ _]
          dyn-events: _ -> [_ _ _ _ _ _ _ _ _ _ _ _ _ _ _ _ _ _]
          timeout: -1 -> [_ _ _ _ _ _ _ _ _ _ _ _ _ _ _ _ _ _]
          tunnel: [_ TRUE _ _ _ _ _ _ _ FALSE _ _ _ _ _ _ _ _] -> w23
          tunnel: w22 -> [w27 w39 w49 w54 w59 w63 w68 w72 w79 w85 w90 w95 w100 w105 w110 w115 w120 w125]
          tunnel: [_ w43 w48 w53 w58 w61 w66 w71 _ w84 w89 w94 w98 w103 w108 w113 w118 w123] -> w21
          tunnel: w20 -> [w26 w42 w47 w52 w57 w62 w67 w73 w78 w82 w88 w93 w99 w104 w109 w114 w119 w124]
          tunnel: [w25 w41 w46 w51 _ w60 w65 w70 _ w83 w87 w92 w97 w102 w107 w112 w117 w122] -> w19
          tunnel: [_ _ _ _ _ _ _ _ w77 _ _ _ _ _ _ _ _ _] -> _
          tunnel: [_ _ _ _ _ _ _ _ w76 _ _ _ _ _ _ _ _ _] -> _
          tunnel: [w24 _ _ _ _ _ _ _ _ _ _ _ _ _ _ _ _ _] -> _
          tunnel: [_ _ _ _ w56 _ _ _ _ _ _ _ _ _ _ _ _ _] -> _
          event Timeout {
            n469 = event-data() -> ()  [unwired: 1 in, 2 out]
            n470 = First Call?() -> (First Call?: T/F=w28:bool)
            n471 = case shown="True" w28 {
              tunnel: w26 -> [w31 w37]
              tunnel: w27 -> [w33 w38]
              tunnel: [w30 w36] -> w25
              tunnel: [w32 w35] -> w24
              frame False {
                n472 = Enqueue Element(queue=w33, element="idle", error in (no error)=w31) -> (queue out=w32:refnum<queue>, error out=w30:errorcluster)  [unwired: 1 in, 1 out]
              }
              frame True {
                n473 = Enqueue Element(queue=w38, element="load file manual", error in (no error)=w37) -> (queue out=w35:refnum<queue>, error out=w36:errorcluster)  [unwired: 1 in, 1 out]
              }
            }
          }
          event "stop": Value Change {
            n474 = event-data() -> ()  [unwired: 1 in, 5 out]
            n475 = Enqueue Element(queue=w39, element="stop", error in (no error)=w42) -> (queue out=w43:refnum<queue>, error out=w41:errorcluster)  [unwired: 1 in, 1 out]
          }
          event "StartRaw": Value Change {
            n476 = event-data() -> ()  [unwired: 1 in, 5 out]
            n477 = Enqueue Element(queue=w49, element="start raw", error in (no error)=w47) -> (queue out=w48:refnum<queue>, error out=w46:errorcluster)  [unwired: 1 in, 1 out]
          }
          event "load file": Value Change {
            n478 = event-data() -> ()  [unwired: 1 in, 5 out]
            n479 = Enqueue Element(queue=w54, element="load file manual", error in (no error)=w52) -> (queue out=w53:refnum<queue>, error out=w51:errorcluster)  [unwired: 1 in, 1 out]
          }
          event "Die Number": Value Change {
            n480 = event-data() -> ()  [unwired: 1 in, 5 out]
            n481 = Enqueue Element(queue=w59, element="Die number picked", error in (no error)=w57) -> (queue out=w58:refnum<queue>, error out=w56:errorcluster)  [unwired: 1 in, 1 out]
          }
          event "Move to": Value Change {
            n482 = event-data() -> ()  [unwired: 1 in, 5 out]
            n483 = Enqueue Element(queue=w63, element="moveto", error in (no error)=w62) -> (queue out=w61:refnum<queue>, error out=w60:errorcluster)  [unwired: 1 in, 1 out]
          }
          event "Move to 0 0": Value Change {
            n484 = event-data() -> ()  [unwired: 1 in, 5 out]
            n485 = Enqueue Element(queue=w68, element="movetofirst", error in (no error)=w67) -> (queue out=w66:refnum<queue>, error out=w65:errorcluster)  [unwired: 1 in, 1 out]
          }
          event "Manual_Test": Value Change {
            n486 = event-data() -> ()  [unwired: 1 in, 5 out]
            n487 = Enqueue Element(queue=w72, element="manual test", error in (no error)=w73) -> (queue out=w71:refnum<queue>, error out=w70:errorcluster)  [unwired: 1 in, 1 out]
          }
          event "J set A/cm2": Value Change {
            n488 = event-data() -> ()  [unwired: 1 in, 5 out]
            n489 = Enqueue Element(queue=w79, element="Jset change", error in (no error)=w78) -> (queue out=w77:refnum<queue>, error out=w76:errorcluster)  [unwired: 1 in, 1 out]
          }
          event "Reset xy": Value Change {
            n490 = event-data() -> ()  [unwired: 1 in, 5 out]
            n491 = Enqueue Element(queue=w85, element="reset xy", error in (no error)=w82) -> (queue out=w84:refnum<queue>, error out=w83:errorcluster)  [unwired: 1 in, 1 out]
          }
          event "Reset 1st die": Value Change {
            n492 = event-data() -> ()  [unwired: 1 in, 5 out]
            n493 = Enqueue Element(queue=w90, element="reset to 1st die", error in (no error)=w88) -> (queue out=w89:refnum<queue>, error out=w87:errorcluster)  [unwired: 1 in, 1 out]
          }
          event "Manual IV settting": Value Change {
            n494 = event-data() -> ()  [unwired: 1 in, 5 out]
            n495 = Enqueue Element(queue=w95, element="change plot", error in (no error)=w93) -> (queue out=w94:refnum<queue>, error out=w92:errorcluster)  [unwired: 1 in, 1 out]
          }
          event "update wafer": Value Change {
            n496 = event-data() -> ()  [unwired: 1 in, 5 out]
            n497 = Enqueue Element(queue=w100, element="update wafer", error in (no error)=w99) -> (queue out=w98:refnum<queue>, error out=w97:errorcluster)  [unwired: 1 in, 1 out]
          }
          event "Select": Value Change {
            n498 = event-data() -> ()  [unwired: 1 in, 5 out]
            n499 = Enqueue Element(queue=w105, element="select", error in (no error)=w104) -> (queue out=w103:refnum<queue>, error out=w102:errorcluster)  [unwired: 1 in, 1 out]
          }
          event "StartFine": Value Change {
            n500 = event-data() -> ()  [unwired: 1 in, 5 out]
            n501 = Enqueue Element(queue=w110, element="start fine", error in (no error)=w109) -> (queue out=w108:refnum<queue>, error out=w107:errorcluster)  [unwired: 1 in, 1 out]
          }
          event "Mask File Raw": Value Change {
            n502 = event-data() -> ()  [unwired: 1 in, 5 out]
            n503 = Enqueue Element(queue=w115, element="raw mask updated", error in (no error)=w114) -> (queue out=w113:refnum<queue>, error out=w112:errorcluster)  [unwired: 1 in, 1 out]
          }
          event "Mask File Manual": Value Change {
            n504 = event-data() -> ()  [unwired: 1 in, 5 out]
            n505 = Enqueue Element(queue=w120, element="mask manual update", error in (no error)=w119) -> (queue out=w118:refnum<queue>, error out=w117:errorcluster)  [unwired: 1 in, 1 out]
          }
          event "Load raw": Value Change {
            n506 = event-data() -> ()  [unwired: 1 in, 5 out]
            n507 = Enqueue Element(queue=w125, element="load raw data", error in (no error)=w124) -> (queue out=w123:refnum<queue>, error out=w122:errorcluster)  [unwired: 1 in, 1 out]
          }
        }
      }
      n508 = Release Queue(queue=w17, force destroy? (F)=TRUE, error in (no error)=w8) -> (error out=→"error out":errorcluster)  [unwired: 2 out]
    }
  }
